vi "ControlUI_Main.vi"(5 "Splash StatusRef":refnum<vi>, 7 "Splash VI Ref":refnum<vi>, 10 "Application":refnum<class "Application.lvclass">, 11 "Main.lvclass":refnum<class "Main.lvclass">) -> ()   [LabVIEW 2019, in "Main.lvclass"]
doc: "Developed by Kevin Thompson\nkevin@thompsonengineering.net\n\nCopyright 2018\nThompson Engineering, LLC"
uses:
  Main.lvclass
  Application/Application.lvclass
  Common/DataTypes/Measurement Config--cluster.ctl
  support/Data Algorithms/subvis/DataTypes/ESR scaling--cluster.ctl
  Common/DataTypes/Acquisition Mode--cluster.ctl
  support/Data Algorithms/subvis/DataTypes/Gain control.ctl
  DataTypes/ESR values--cluster.ctl
  <vilib>/userDefined/High Color/nirio_resource_hc.ctl
  DataTypes/Control UI - AppData--cluster.ctl
  DataTypes/Settings--cluster.ctl
  DataTypes/Dependency--cluster.ctl
  Config/Config.lvclass
  DAQ_Engine/DAQ_Engine.lvclass
  Log_Engine/Log_Engine.lvclass
  DataTypes/Public Events--cluster.ctl
  Common/DataTypes/TD Async CmdMsg EventData--cluster.ctl
  Common/DataTypes/UpdateControlValue EvData--cluster.ctl
  DataTypes/ProcessingStateChg EvData--cluster.ctl
  DataTypes/ProcessingState--enum.ctl
  Common/DataTypes/InverterWaveforms--QRef.ctl
  Common/DataTypes/InverterWaveforms--cluster.ctl
  Common/DataTypes/ChannelWaveforms--cluster.ctl
  Common/DataTypes/DataProcAuxDat--Qref.ctl
  DataTypes/DataProcessAuxData--cluster.ctl
  <vilib>/TELLC/Dynamic CVT API/TD Dynamic CVT DVR--ref.ctl
  Common/DataTypes/TD GetSet ActionSelect--enum.ctl
  Main.lvclass/Main.ctl
  DAQ_Engine/DataTypes/AsynCmd_DAQ_Engine--enum.ctl
  DataTypes/PrivateAsynEv_Main--enum.ctl
  DataTypes/AsynMsg_Main--enum.ctl
  DataTypes/InverterInfo--cluster.ctl
  DataTypes/StartProcInitParams--cluster.ctl
  DataTypes/ProcessInitParams--cluster.ctl
  Common/DataTypes/DAQState--enum.ctl
  Common/DataTypes/LogState--enum.ctl
  Common/DataTypes/TDMSState--enum.ctl
  Log_Engine/Log_Engine.lvclass/Log_Engine.ctl
  DAQ_Engine/DAQ_Engine.lvclass/DAQ_Engine.ctl
  Application/DataTypes/AsynMsg_Application--enum.ctl
  Common/DataTypes/Inverter database record v2--cluster.ctl
  Common/DataTypes/inverter info v2--cluster.ctl
  Common/DataTypes/inverter gain range--cluster.ctl
  Common/DataTypes/inverter offset range--cluster.ctl
  Accessors/Get Settings.vi
  Accessors/Get PublicEvents.vi
  Accessors/Get Dependency.vi
  Accessors/Get TerminateAppEvent.vi
  Accessors/Get InvWfms-DT-QRef.vi
  Accessors/Get DPAuxData-QRef.vi
  Accessors/Get InverterLUT Dict Ref.vi
  Accessors/Get CurrInverter Record.vi
  Accessors/Set CurrInverter Record.vi
  Accessors/Get ObjData.vi
  Log_Engine/Accessors/Get PublicEvents.vi
  DAQ_Engine/Accessors/Get PublicEvents.vi
  DAQ_Engine/Accessors/Get MeasSettings.vi
  DAQ_Engine/Accessors/Get Settings.vi
  <userlib>/_OpenG.lib/comparison/comparison.llb/String Changed__ogtk.vi
  <vilib>/TELLC/SMQ/Add States to Queue using MultiLine String with vData.vi
  <userlib>/_OpenG.lib/error/error.llb/Filter Error Codes (Array)__ogtk.vi
  Common/Startup/GBL System.vi
panel:
  in  "Acqusition Mode":T1
  in  "Trigger SelectInverter Event":bool
  in  "LeftPanelTab":T2(tab)=enum."Settings"
  out "InvSelLED":bool
  in  "Selected Inverter":string[](array[string])
  in  "SelectInverter":bool
  in  "Inverter List":i32[](listbox)
  in  "Signal scaling":T3[](array[typedef])
  in  "Degassing rate\n9775":u32=3
  in  "Averaging samples\n9215":u32=480000
  in  "Data Rate 9215\n(S/s)":dbl=1200000.0 format="%#.6p"
  in  "Data Rate 9775\n(S/s)":dbl=3.0 format="%#.6p"
  out "DAQEnabled":bool=TRUE
  in  "DAQEnDis":bool
  out "LogEnabled":bool
  in  "LogEnDis":bool
  out "TDMSEnabled":bool
  in  "TDMSEnDis":bool
  in  "StopProcessing":bool caption="StopProcess"
  out "Processing":bool=TRUE
  in  "StartProcessing":bool caption="StartProcess"
  in  "UpdateDAQSettings":bool
  in  "cRIO Error\nReporting Mode":i32(ring) items=["DONTPRINT", "PRINTWARNINGS", "PRINTFATAL", "PRINTALL"]
  in  "NumPF RdsToAvg":i32=2 caption="Number PF\nReads to Avg"
  in  "ESR alarm threshhold (%)":dbl=200.0
  in  "# readings to average":i32=40
  in  "RIO Device":T4
  out "DP AuxData Size":i32
  out "InvWfmsQ DT size":i32
  in  "Inverter ID":string
  in  "toggle scrollbars":bool
  in  "toggle MainTabDbgPg":bool
  out "DAQ Running":bool=TRUE
  out "MeasSet":T5={"Data Rate 9775"=3.0, "Data Rate 9215"=1200000.0, "Samples RMS 9215"=480000, "Samples RMS 9775"=3}
  out "DAQError":bool caption="DAQ Error"
  in  "SystemError":bool
  out "Sel_PowerFactor_Data":bool=TRUE
  in  "Show_PowerFactor_Data":bool
  out "Sel_TimeSeries_Data":bool
  in  "Show_TimeSeries_Data":bool
  out "Sel_ESR_Data":bool
  in  "Show_ESR_Data":bool
  in  "MainPanelTab":T6(tab)=enum."PowerFactorData"
  in  "StoreESR BLine":bool
  in  "UseSavedESR BLine":bool
  in  "set alarm":bool
  in  "reset averaging":bool
  in  "reset alarm":bool
  in  "ESR scaling":T7[](array[typedef]) caption="ESR scaling\n(manual adjustment)" {"Offset" format="%^#_6g"; "Gain" format="%^#_6g"}
  in  "Tab Control":enum32{"DUT1", "DUT2", "DUT3", "DUT4"}(tab)
  out "ESR values 1":T8 caption="ESR values" {"Scaled & avgd ESR" format="%_4e"; "Max ESR" format="%_4e"; "Raw  ESR" format="%.3e"}
  out "Equivalent Series Resistance (ESR) 1":T9(graph)
  in  "MinCurrThreshold 1":dbl=1.5 caption="Minimum Current\nThreshold (A)" format="%.8f"
  in  "Sensor Type 1":i32(ring)
  in  "Sensor Type 2":i32(ring)
  in  "MinCurrThreshold 2":dbl=1.5 caption="Minimum Current\nThreshold (A)" format="%.8f"
  out "ESR values 2":T8 caption="ESR values" {"Scaled & avgd ESR" format="%_4e"; "Max ESR" format="%_4e"; "Raw  ESR" format="%.3e"}
  out "Equivalent Series Resistance (ESR) 2":T9(graph)
  in  "Sensor Type 3":i32(ring)
  in  "MinCurrThreshold 3":dbl=1.5 caption="Minimum Current\nThreshold (A)" format="%.8f"
  out "ESR values 3":T8 caption="ESR values" {"Scaled & avgd ESR" format="%_4e"; "Max ESR" format="%_4e"; "Raw  ESR" format="%.3e"}
  out "Equivalent Series Resistance (ESR) 3":T9(graph)
  in  "Sensor Type 4":i32(ring)
  in  "MinCurrThreshold 4":dbl=1.5 caption="Minimum Current\nThreshold (A)" format="%.8f"
  out "ESR values 4":T8 caption="ESR values" {"Scaled & avgd ESR" format="%_4e"; "Max ESR" format="%_4e"; "Raw  ESR" format="%.3e"}
  out "Equivalent Series Resistance (ESR) 4":T9(graph)
  out "Iout 60Hz":waveform(dbl)[](graph)
  out "Iout ripple":waveform(dbl)[](graph)
  out "Iin ripple":waveform(dbl)[](graph)
  out "DUT4 I-V":waveform(dbl)[](graph) caption="DUT 4"
  out "DUT3 power data":T10 caption="Phase 1" {"Vout (RMS)" format="%0.2f"; "Iout (RMS)" format="%0.2f"; "PF" format="%.3g"}
  out "DUT2 power data":T10 caption="Phase 1" {"Vout (RMS)" format="%0.2f"; "Iout (RMS)" format="%0.2f"; "PF" format="%.3g"}
  out "DUT3 I-V":waveform(dbl)[](graph) caption="DUT 3"
  out "DUT2 I-V":waveform(dbl)[](graph) caption="DUT 2"
  out "DUT1 I-V":waveform(dbl)[](graph) caption="DUT 1"
  out "DUT1 power data":T10 caption="Phase 1" {"Vout (RMS)" format="%0.2f"; "Iout (RMS)" format="%0.2f"; "PF" format="%.3g"}
  in  "Dummy Vrms":dbl format="%.2g"
  in  "UseDummyVrms":bool
  out "DUT4 power data":T10 caption="Phase 1" {"Vout (RMS)" format="%0.2f"; "Iout (RMS)" format="%0.2f"; "PF" format="%.3g"}
  in  "Page2Pg_button":bool
  in  "SettingsPg_button":bool
  in  "DataPg_button":bool
  in  "ConfigPg_button":bool
  in  "Exit":bool
  in  "TitleBar AppVerText":string="v2.0.2 build-003"
  in  "TitleBar Text":string="INVERTER   HEALTH   SCANNER   SYSTEM"
  in  "TitleBar":bool
  in  "StatusMsg":string caption="Status"
  in  "process sync":refnum<notifier>
  # "click to reset"
  # "Run Time Data Panel"
  # "Inverter Selection"
  # "right-click to open table editor"
  # "Configuration Panel"
  # "Gain"
  # "Offset"
  # "Iin ripple"
  # "Iout ripple"
  # "Iout 60Hz"
  # "Vout 60"
  # "Settings Panel"
  # "Ripple Current"
  # "RMS & Power Factor"
  # "ESR Data"
  # "Gain"
  # "Offset"
  # "Time Series Data"
  # "DUT 1"
  # "DUT 2"
  # "DUT 3"
  # "DUT 4"
  # "Power Factor Data - Phase Current and Voltage"
  # "DUT 3"
  # "DUT 2"
  # "DUT 1"
  # "Current (A)"
  # "Voltage (V)"
  # "DUT 4"
  # "Debug Page"
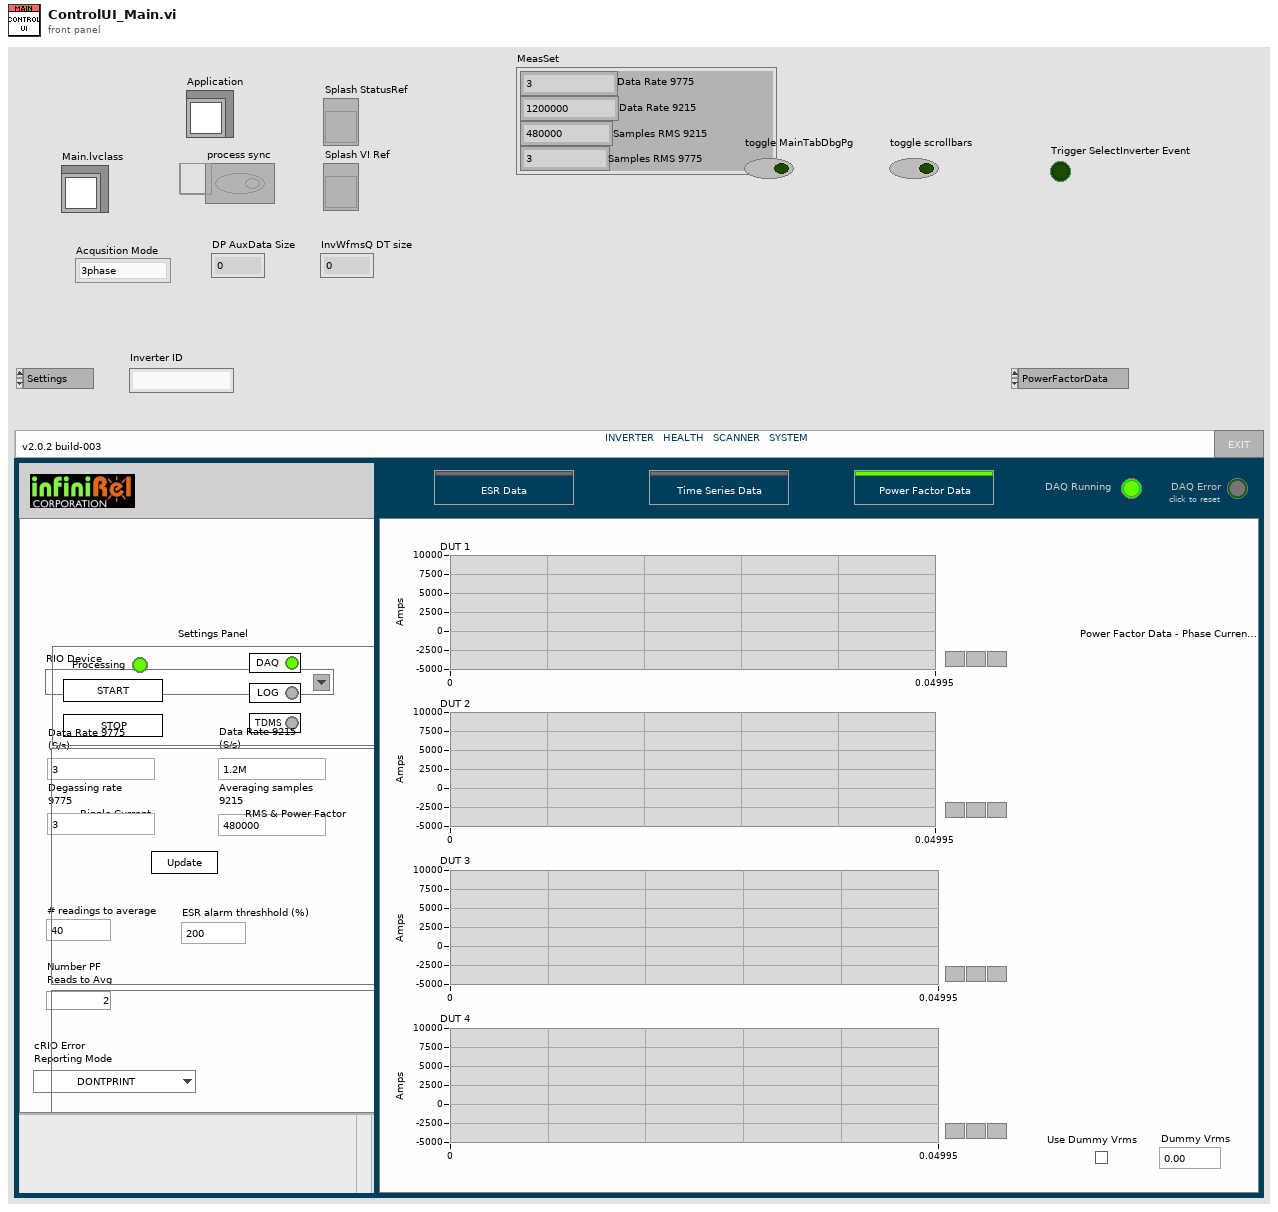
[diagram p1: front panel]
types:
  T1 = typedef "Acquisition Mode--cluster.ctl" = enum16{"3phase", "Single"}
  T2 = enum32{"Data", "InverterSel", "Config", "Settings"}
  T3 = typedef "Main.lvclass/Gain control.ctl" = cluster{"Iin ripple gain":dbl, "Iout ripple gain":dbl, "Iout 60Hz gain ":dbl, "Vout 60Hz gain ":dbl, "Iin ripple offest":dbl, "Iout ripple offset":dbl, "Iout 60Hz offset":dbl, "Vout 60Hz offset":dbl}
  T4 = typedef "nirio_resource_hc.ctl" = tag
  T5 = typedef "Measurement Config--cluster.ctl" = cluster{"Data Rate 9775":dbl, "Data Rate 9215":dbl, "Samples RMS 9215":u32, "Samples RMS 9775":u32}
  T6 = enum32{"ESRData", "TimeSeriesData", "PowerFactorData", "DebugPage"}
  T7 = typedef "Main.lvclass/ESR scaling--cluster.ctl" = cluster{"Gain":dbl, "Offset":dbl}
  T8 = typedef "Main.lvclass/ESR values--cluster.ctl" = cluster{"Inverter State":string, "Raw  ESR":dbl, "Max ESR":dbl, "Scaled & avgd ESR":dbl, "Inverter ESR status":bool}
  T9 = cluster{"ESR Baseline":dbl, "Alarm threshhold (%)":dbl, "Avg value":dbl}
  T10 = cluster{"PF":dbl, "Iout (RMS)":dbl, "Vout (RMS) ":dbl, "Power (W)":dbl}
  T11 = typedef "Main.lvclass/ProcessingState--enum.ctl" = enum16{"Idle", "Starting", "Running", "Done", "Error"}
  T12 = typedef "TD GetSet ActionSelect--enum.ctl" = enum16{"Init", "Get", "Set"}
  T13 = typedef "Main.lvclass/Control UI - AppData--cluster.ctl" = cluster{"Core":cluster{"Current VI Reference":refnum<vi>, "Close Panel on Exit?":bool}, "SMQ":refnum<queue>, "Initialized?":bool, "Self Reference":refnum<class "Main.lvclass">, "Simulation?":bool, "process sync":refnum<notifier>, "vData":variant, "Settings":T14, "Dependency":T15, "Public Events":T16, "Splash StatusRef":refnum<vi>, "Splash VI Ref":refnum<vi>, "RunTimeSystem?":bool, "StatusMsg Ref":refnum<vi>, "AppTerminateEv":refnum<user-event>, "MenuRef":refnum<k9>, "DAQEnabled":bool, "LoggingEnabled":bool, "TDMS Enabled":bool, "Application":refnum<class "Application.lvclass">, "InvWfmsQ-DT":T17, "DPAuxDataQ":T18, "ProcessingState":T11, "DisplayLoopInterval":u32, "MenuBarShown?":bool, "InverterNames[]":string[], "InverterLUT Dict":T19}
  T14 = typedef "Main.lvclass/Settings--cluster.ctl" = cluster{"Simulation":bool, "Signal scaling":T3[], "ESR scaling":T7[], "num readings to average":i32[], "ESR alarm threshhold (%)":i32[], "UseDummyVrms":bool, "Dummy Vrms":dbl, "Inverter Database File":path, "default Inverter (name)":string[], "Minimum Current Threshold ":dbl[], "Sensors Database File":path, "default Sensors (name)":string[]}
  T15 = typedef "Main.lvclass/Dependency--cluster.ctl" = cluster{"Config":refnum<class "Config.lvclass">, "DAQ":refnum<class "DAQ_Engine.lvclass">, "Log_Engine":refnum<class "Log_Engine.lvclass">}
  T16 = typedef "Main.lvclass/Public Events--cluster.ctl" = cluster{"Main.AsyncCmd Event":refnum<user-event>, "Main.AsyncMsg Event":refnum<user-event>, "stop process":refnum<user-event>, "UpdateControlValue Ev":refnum<user-event>, "ProcessingStateChg Ev":refnum<user-event>}
  T17 = typedef "InverterWaveforms--QRef.ctl" = refnum<queue>
  T18 = typedef "DataProcAuxDat--Qref.ctl" = refnum<queue>
  T19 = typedef "TD Dynamic CVT DVR--ref.ctl" = refnum<data-value>
  T20 = cluster{"AvgPF":dbl, "IoutRMS_A":dbl, "VoutRMS_V":dbl, "Power_W":dbl}
  T21 = typedef "DataProcessAuxData--cluster.ctl" = cluster{"Time Stamp":timestamp, "Raw ESR sum":dbl, "Inv 1 ON?":bool, "Average scaled ESR sum":dbl, "Inv 1 over threshold?":bool, "Inv 1 ESR":cluster{"ESR Baseline":dbl, "Alarm threshhold (%)":dbl, "Avg value":dbl}, "Max ESR":dbl}
  T22 = cluster{"Inverter 1 state: ":string, "Raw ESR sum":dbl, "Max ESR":dbl, "Average scaled ESR sum":dbl, "Inv 1 over threshold?":bool}
  T23 = typedef "InverterWaveforms--cluster.ctl" = T24[]
  T24 = typedef "ChannelWaveforms--cluster.ctl" = cluster{"Iin ripple ":waveform(dbl), "Iout ripple ":waveform(dbl), "Iout 60Hz":waveform(dbl), "Vout 60Hz":waveform(dbl)}
  T25 = typedef "DAQ_Engine.lvclass/AsynCmd_DAQ_Engine--enum.ctl" = enum16{"DAQ.EnableDAQ", "DAQ.ClearDAQError", "DAQ.SetMeasConfig", "DAQ.SetAcqMode", "DAQ.SetErrorReporting"}
  T26 = typedef "Main.lvclass/PrivateAsynEv_Main--enum.ctl" = enum16{"PrivMain.UpdateMeasSettings", "PrivMain.UpdateAcqMode", "PrivMain.UpdateDAQState", "PrivMain.UpdateLogState", "PrivMain.UpdateTDMSState", "PrivMain.UpdateProcessingState", "PrivMain.Stop&Terminate", "PrivMain.CurrInverterUpdated", "PrivMain.UpdateStoreUseESRBaseline", "PrivMain.SetUnsetAlarm&ESRBLine", "PrivMain.ResetAveraging"}
  T27 = typedef "Main.lvclass/AsynMsg_Main--enum.ctl" = enum16{"Main.CurrInverterUpdated"}
  T28 = typedef "Main.lvclass/StartProcInitParams--cluster.ctl" = cluster{"InverterInfo":T29[], "ProcessInitParams":T30[]}
  T29 = typedef "InverterInfo--cluster.ctl" = cluster{"Inverter ID":string}
  T30 = typedef "Main.lvclass/ProcessInitParams--cluster.ctl" = cluster{"MinCurrThreshold":dbl, "NumPF RdsToAvg":i32, "ESR alarm threshhold (%)":dbl, "# readings to average":i32}
  T31 = typedef "DAQState--enum.ctl" = enum16{"Unknown", "Stopped", "Running", "Error"}
  T32 = cluster{"VoltageDyn":dbl, "CurrentDyn":dbl, "MotorV SP":dbl}[]
  T33 = enum32{"invalid app kind", "Development System", "Run Time System", "Student Edition", "Embedded LabVIEW", "Evaluation", "Custom"}
  T34 = typedef "Application.lvclass/AsynMsg_Application--enum.ctl" = enum16{"Application.AppClassReference"}
  T35 = enum16{"Left Button", "Center Button", "Right Button", "Window Close"}
  T36 = enum32{"Invalid", "Standard", "Closed", "Hidden", "Minimized", "Maximized"}
  T37 = enum32{"Invalid", "Default", "Floating", "Floating/Auto-Hide", "Modal"}
  T38 = typedef "Inverter database record v2--cluster.ctl" = cluster{"name":string, "last updated":timestamp, "type":string, "inverter Info":T39, "gain range":T40, "offset range":T41, "gain actual":dbl, "offset actual":dbl, "power level":dbl, "minimum current":dbl, "resistance single phase":dbl, "resistance 3 phase":dbl, "set flag":u16}
  T39 = typedef "inverter info v2--cluster.ctl" = cluster{"manufacturer":string, "model":string, "product":string, "serial":string, "power class":string, "year manf":string}
  T40 = typedef "inverter gain range--cluster.ctl" = cluster{"gain max":dbl, "gain min":dbl, "gain increment":dbl}
  T41 = typedef "inverter offset range--cluster.ctl" = cluster{"offset max":dbl, "offset min":dbl, "offset increment":dbl}
  T42 = typedef "Config.lvclass/Config Settings.ctl" = cluster{"Application Settings":T43, "Main Settings":T14, "DAQ Settings":T44, "LogEngine Settings":T45}
  T43 = typedef "Application.lvclass/Settings--cluster.ctl" = cluster{"Simulation":bool}
  T44 = typedef "DAQ_Engine.lvclass/Settings--cluster.ctl" = cluster{"Simulation":bool, "Initial ErrReporting setting":i32, "Initial Measurement settings":T5, "Acquisition mode":T1, "DemoMode":bool, "RIO Device":string}
  T45 = typedef "Log_Engine.lvclass/Settings--cluster.ctl" = cluster{"Simulation":bool, "TDMS_FolderPath":string, "CSV_FolderPath":string, "TDMS_FileName_Prefix":string, "CSV_FileName_Prefix":string, "TDMS_LogDuration(s)":dbl, "CSV_LogDuration(s)":dbl}
  T46 = typedef "TD Pathnames--cluster.ctl" = cluster{"RunTimeSys?":bool, "AppFolder":path, "ExecutablePath":path, "ConfigFolder":path, "DataLogFolder":path, "SystemLogFolder":path, "SeqFolder":path, "MainStartupPathname":path, "MainUIPathname":path, "SystemEventsFile":path, "SeqEventsFile":path, "Config SettingsFile":path, "DAQ IOConfigFile":path, "SystemSimulation":bool}
  T47 = typedef "DAQ_Engine.lvclass/DAQStateEvData--cluster.ctl" = cluster{"DAQState":T31, "vData":variant}
  T48 = typedef "LogState--enum.ctl" = enum16{"Unknown", "Stopped", "Running", "Error"}
  T49 = typedef "Log_Engine.lvclass/LogStateEvData--cluster.ctl" = cluster{"LogState":T48, "vData":variant}
  T50 = typedef "TDMSState--enum.ctl" = enum16{"Unknown", "Stopped", "Running", "Error"}
  T51 = typedef "Log_Engine.lvclass/TDMSStateEvData--cluster.ctl" = cluster{"TDMSState":T50, "vData":variant}
  T52 = typedef "Main.lvclass/AsynCmd_Main--enum.ctl" = enum16{"Main.StartProcessing", "Main.StopProcessing", "Main.RefreshInverterList"}
  T53 = typedef "Main.lvclass/ObjData--cluster.ctl" = cluster{"Settings":T14, "Public Events":T16, "Dependency":T15, "ReadData-placeholder":T54, "VISA-placeholder":refnum<visa-resource-name>, "InverterWaveformsQ":T17, "Application.TerminateProcess Event":refnum<user-event>, "RawDaqDataQ":T55, "MeasSettings":T5, "InverterDataAcqMode":T1, "DAQState Data":T47, "Private Events":T56, "InvWfmsQ-DT":T17, "DPAuxDataQ":T18, "ProcessingState":T11, "InverterInfo":T29, "CurrInverters":T38[], "InverterLUT Dict":T19, "ESR Chart Ref":refnum<vi>[], "StoreESR BLine Ref":refnum<vi>, "UseSavedESR BLine Ref":refnum<vi>, "CurrSensor":T57, "SensorLUT Dict":T19}
  T54 = typedef "Main.lvclass/Read Data--cluster.ctl" = cluster{"Data":dbl}
  T55 = typedef "RawDAQDataQRef--cluster.ctl" = refnum<queue>
  T56 = typedef "Main.lvclass/Private Events--cluster.ctl" = cluster{"PrivateAsync Ev":refnum<user-event>}
  T57 = typedef "Sensor LUT--cluster.ctl" = T58[]
  T58 = typedef "Sensor database record--cluster.ctl" = cluster{"name":string, "last updated":timestamp, "manufacturer":string, "model":string, "Sensitivity index":dbl, "Sensor Ranges":T59}
  T59 = typedef "Sensor ranges--cluster.ctl" = cluster{"Max.VOut.RMS (V)":dbl, "Max.Out.Peak (V)":dbl, "Sensitivity (mV/A)":dbl, "Max.IOut.RMS(A)":dbl, "Min.IOut.RMS(A)":dbl}
  T60 = typedef "DAQ_Engine.lvclass/Public Events--cluster.ctl" = cluster{"DAQ_Engine.AsyncCmd Event":refnum<user-event>, "DAQ_Engine.AsyncMsg Event":refnum<user-event>, "stop process":refnum<user-event>, "DAQ_Engine.DAQStateChg Ev":refnum<user-event>, "DAQ_Engine.MeasSettingsChg Ev":refnum<user-event>, "DAQ_Engine.AcqModeChg Ev":refnum<user-event>}
  T61 = typedef "Log_Engine.lvclass/Public Events--cluster.ctl" = cluster{"Log_Engine.AsyncCmd Event":refnum<user-event>, "Log_Engine.AsyncMsg Event":refnum<user-event>, "stop process":refnum<user-event>, "Log_Engine.LogStateChg Ev":refnum<user-event>, "Log_Engine.TDMSStateChg Ev":refnum<user-event>}
  T62 = cluster{"Current VI Reference":refnum<vi>, "Close Panel on Exit?":bool}
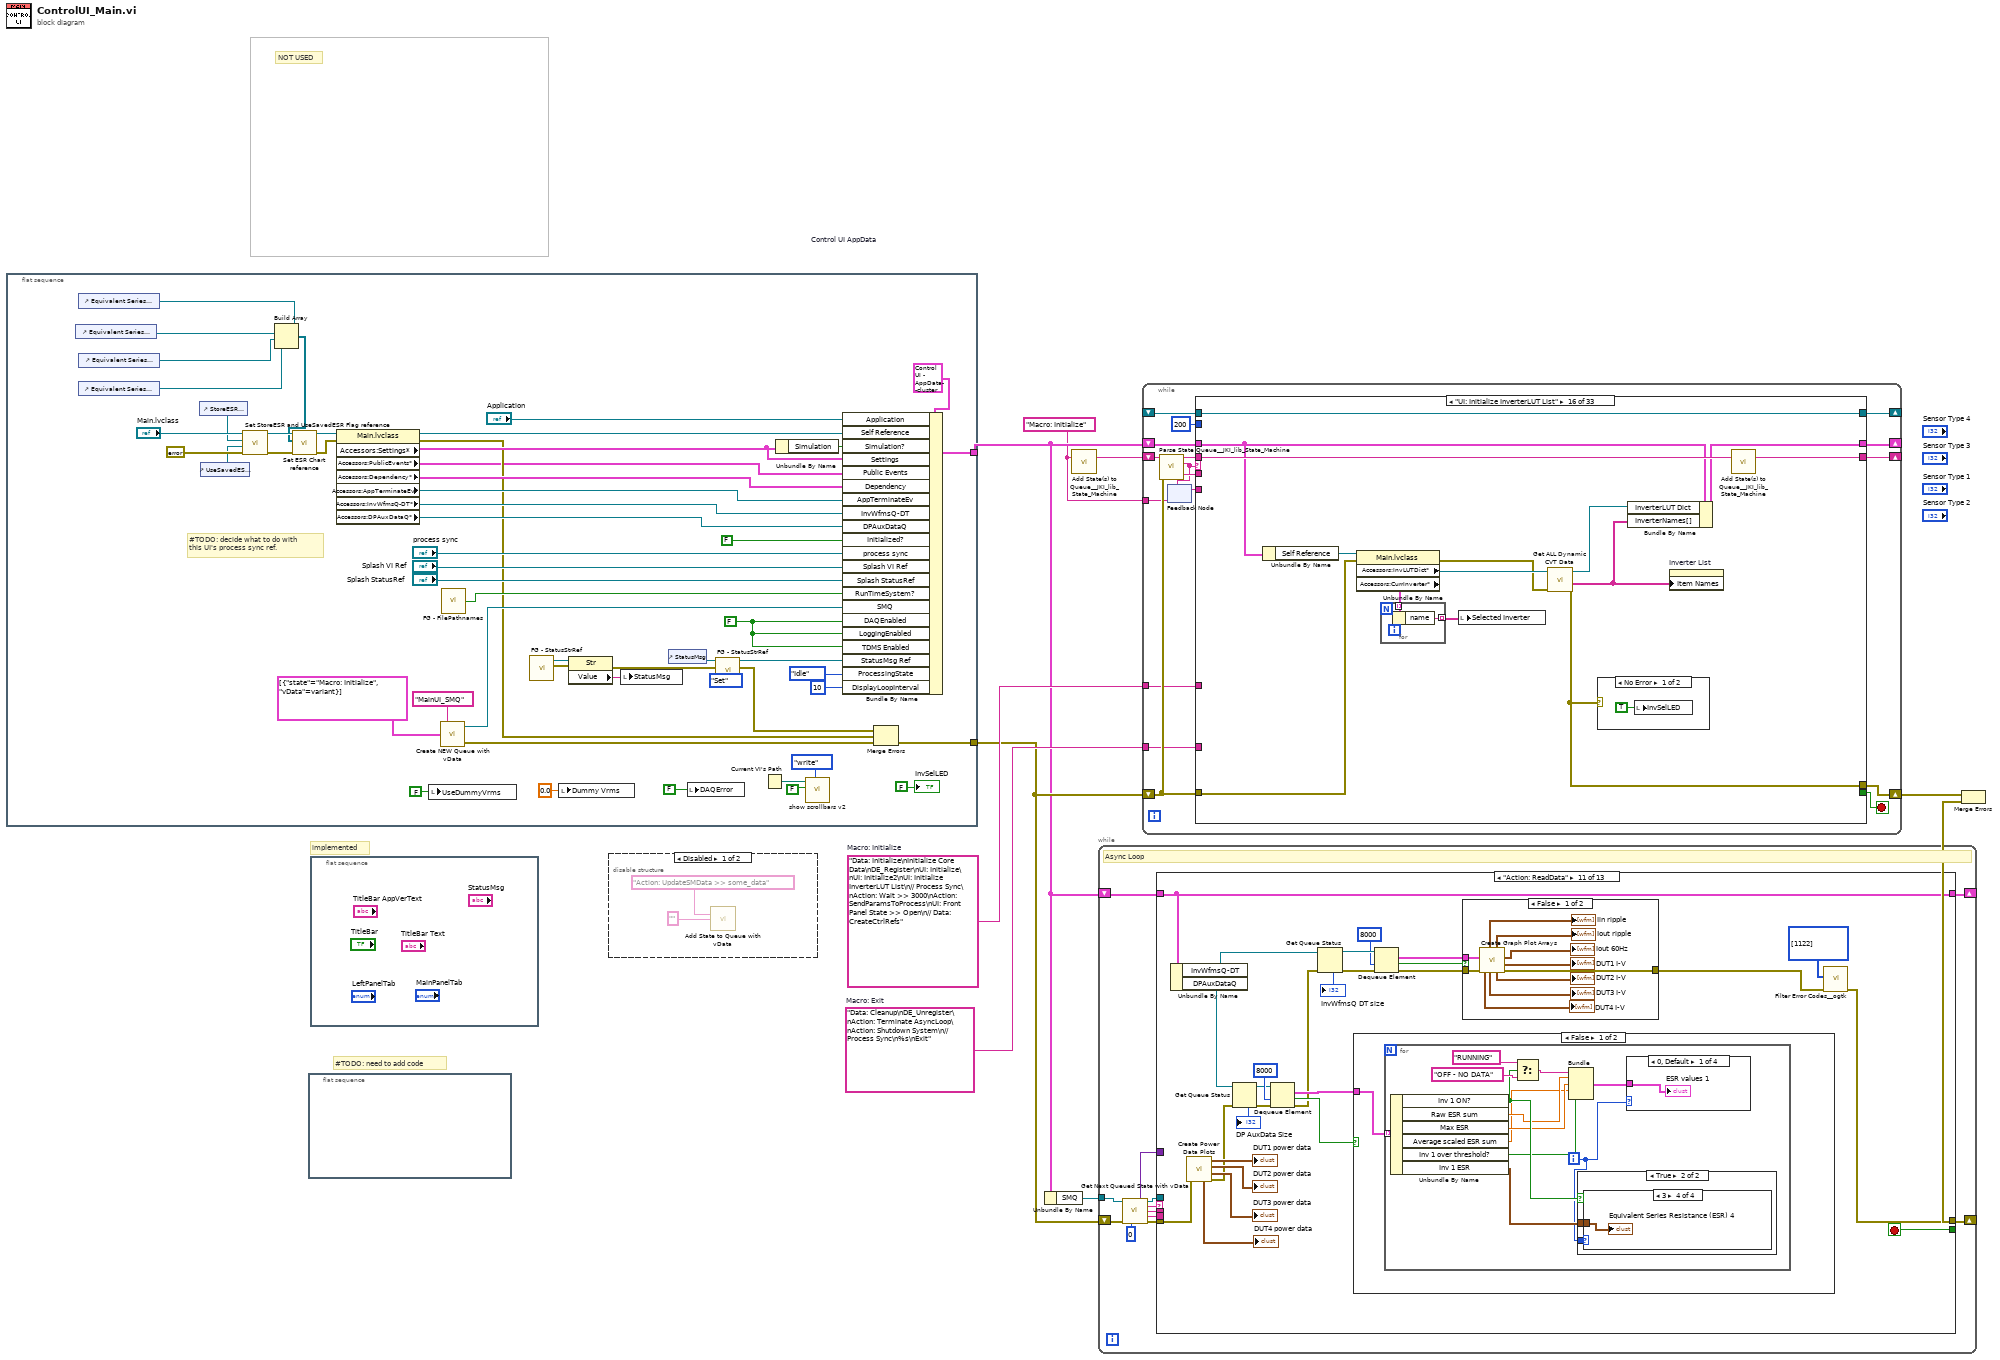
[diagram p0: block diagram]
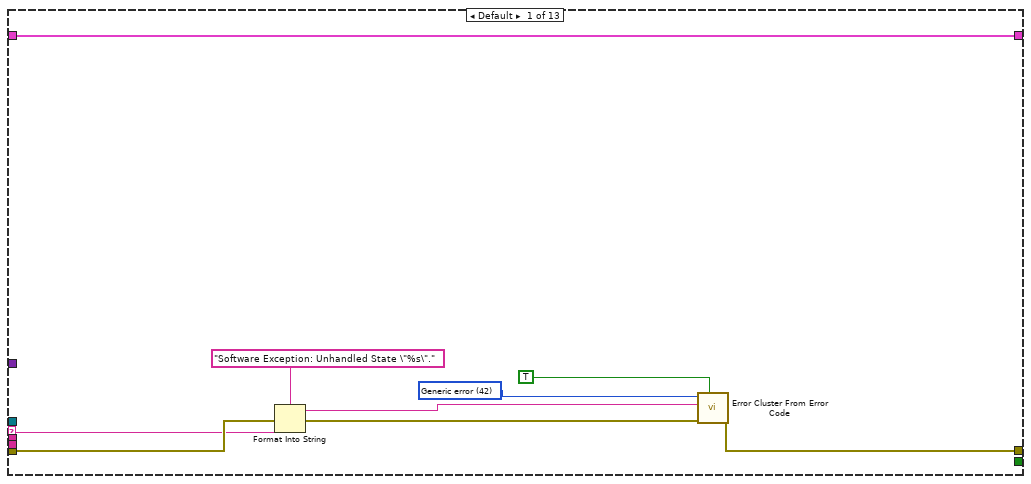
[diagram p3: hidden frame]
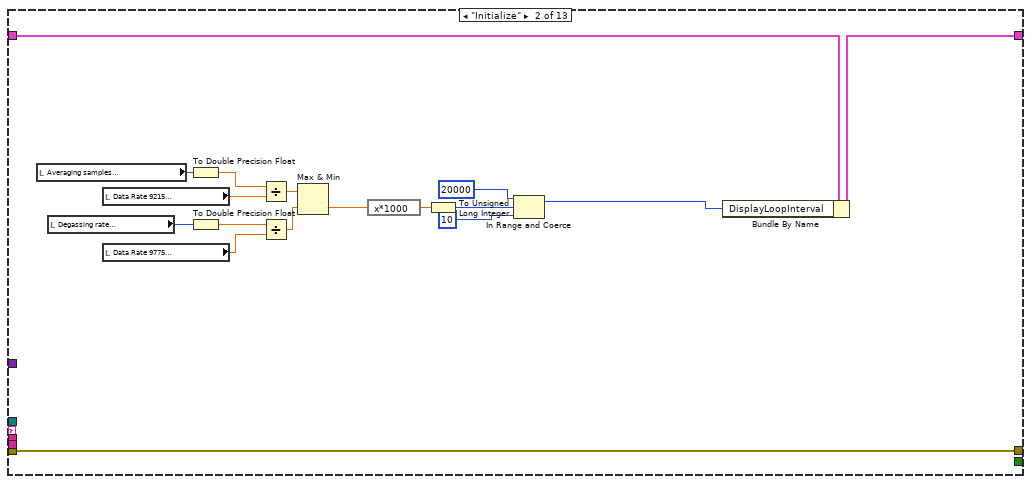
[diagram p4: hidden frame]
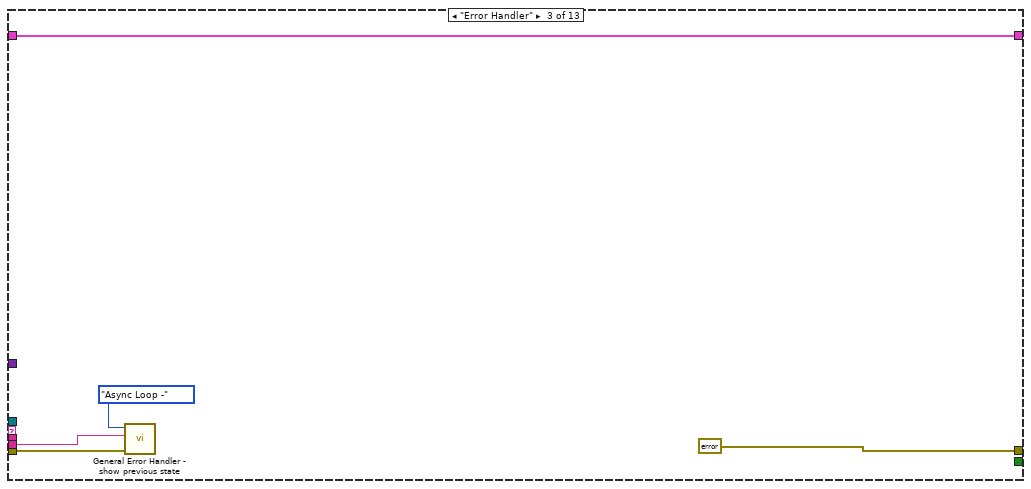
[diagram p5: hidden frame]
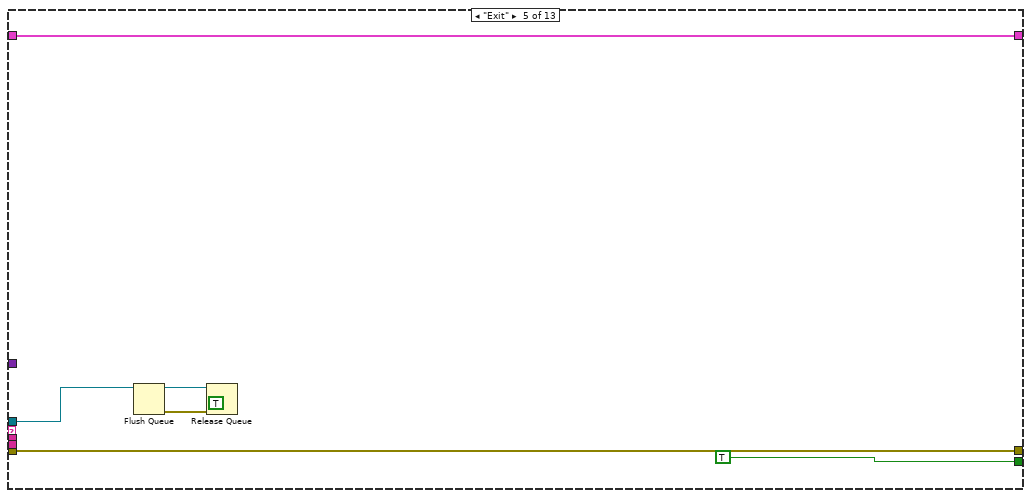
[diagram p7: hidden frame]
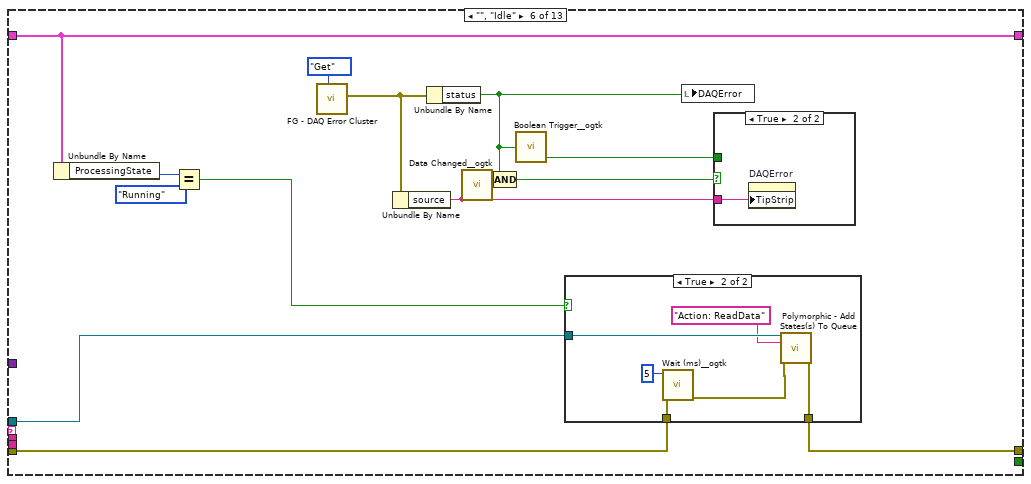
[diagram p8: hidden frame]
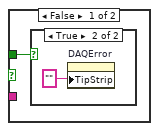
[diagram p9: hidden frame]
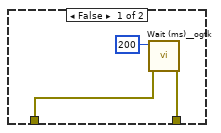
[diagram p11: hidden frame]
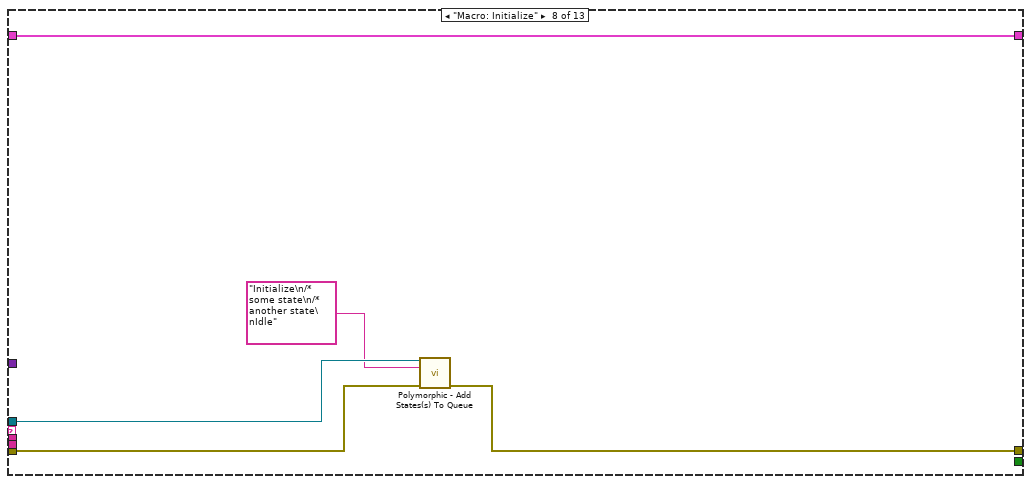
[diagram p13: hidden frame]
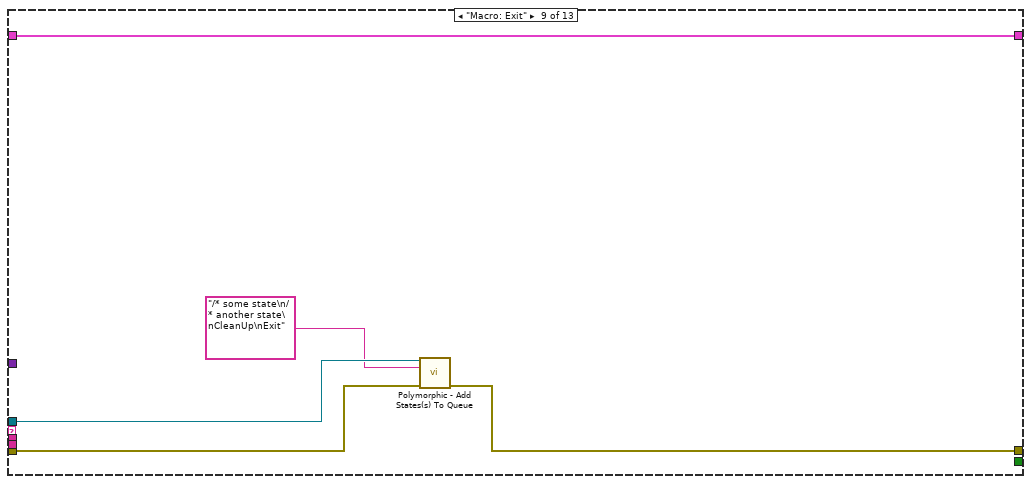
[diagram p14: hidden frame]
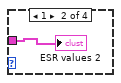
[diagram p16: hidden frame]
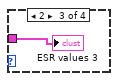
[diagram p17: hidden frame]
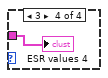
[diagram p18: hidden frame]
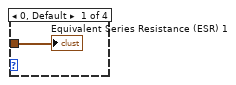
[diagram p20: hidden frame]
diagram:
  w7 = "Data: Cleanup\nDE_Unregister\nAction: Terminate AsyncLoop\nAction: Shutdown System\n// Process Sync\n%s\nExit"  # Macro: Exit
  w8 = "Data: Initialize\nInitialize Core Data\nDE_Register\nUI: Initialize\nUI: Initialize2\nUI: Initialize InverterLUT List\n// Process Sync\nAction: Wait >> 3000\nAction: SendParamsToProcess\nUI: Front Panel State >> Open\n// Data: CreateCtrlRefs"  # Macro: Initialize
  w1 = "Macro: Initialize"
  # "implemented"
  # "#TODO: need to add code"
  # "NOT USED"
  n1 = flat-sequence {
    tunnel: [w62] -> w4
    tunnel: [w47] -> w6
    frame #0 {
      w33 = FALSE
      w54 = T13 {"Core"={"Current VI Reference"=refnum, "Close Panel on Exit?"=FALSE}, "SMQ"=refnum, "Initialized?"=FALSE, "Self Reference"=refnum, "Simulation?"=FALSE, "process sync"=refnum, "vData"=variant, "Settings"={"Simulation"=FALSE, "Signal scaling"=[], "ESR scaling"=[], "num readings to average"=[], "ESR alarm threshhold (%)"=[], "UseDummyVrms"=FALSE, "Dummy Vrms"=0.0, "Inverter Database File"=path "", "default Inverter (name)"=[], "Minimum Current Threshold "=[], "Sensors Database File"=path "", "default Sensors (name)"=[]}, "Dependency"={"Config"=refnum, "DAQ"=refnum, "Log_Engine"=refnum}, "Public Events"={"Main.AsyncCmd Event"=refnum, "Main.AsyncMsg Event"=refnum, "stop process"=refnum, "UpdateControlValue Ev"=refnum, "ProcessingStateChg Ev"=refnum}, "Splash StatusRef"=refnum, "Splash VI Ref"=refnum, "RunTimeSystem?"=FALSE, "StatusMsg Ref"=refnum, "AppTerminateEv"=refnum, "MenuRef"=refnum, "DAQEnabled"=FALSE, "LoggingEnabled"=FALSE, "TDMS Enabled"=FALSE, "Application"=refnum, "InvWfmsQ-DT"=refnum, "DPAuxDataQ"=refnum, "ProcessingState"=enum."Idle", "DisplayLoopInterval"=0, "MenuBarShown?"=FALSE, "InverterNames[]"=[], "InverterLUT Dict"=refnum}  # Control UI AppData
      # "#TODO: decide what to do with\nthis UI's process sync ref."
      n2 = control-ref of="Equivalent Series Resistance (ESR) 2"() -> (w12:refnum<vi>)
      n3 = control-ref of="Equivalent Series Resistance (ESR) 1"() -> (w14:refnum<vi>)
      n4 = control-ref of="Equivalent Series Resistance (ESR) 4"() -> (w10:refnum<vi>)
      n5 = control-ref of="Equivalent Series Resistance (ESR) 3"() -> (w11:refnum<vi>)
      n6 = control-ref of="StoreESR BLine"() -> (w15:refnum<vi>)
      n7 = control-ref of="UseSavedESR BLine"() -> (w16:refnum<vi>)
      n8 = call "Set StoreESR and UseSavedESR Flag reference.vi"("error in (no error)"=errorcluster {"status"=FALSE, "code"=0, "source"=""} ("error constant"), "UseSavedESR BLine Ref"=w16, "StoreESR BLine Ref"=w15, "Main in"="Main.lvclass") -> ("error out"=w19:errorcluster, "Main out"=w20:refnum<class "Main.lvclass">)  [unwired: 6 in]
      n9 = Build Array(w14, w12, w11, w10) -> (w13:refnum<vi>[])
      n10 = call "Set ESR Chart reference.vi"("error in (no error)"=w19, "ESR Chart Ref"=w13, "Main in"=w20) -> ("error out"=w17:errorcluster, "Main out"=w22:refnum<class "Main.lvclass">)  [unwired: 7 in]
      n11 = property class="Main.lvclass"(reference=w22, error in=w17) -> (reference out=w25:refnum<class "Main.lvclass">, error out=w26:errorcluster, "Accessors:Settings*"=w56:T14, "Accessors:PublicEvents*"=w24:T16, "Accessors:Dependency*"=w58:T15, "Accessors:AppTerminateEv*"=w53:refnum<user-event>, "Accessors:InvWfmsQ-DT*"=w32:T17, "Accessors:DPAuxDataQ*"=w31:T18)
      n12 = local write "UseDummyVrms"(FALSE ("UseDummyVrms")) -> ()
      n13 = call <vilib>:"Create NEW Queue with vData.vi"("Initial States"=cluster{"state":string, "vData":variant}[] [{"state"="Macro: Initialize", "vData"=variant}], "Name (SMQ)"="MainUI_SMQ") -> ("error out"=w48:errorcluster, "queue out"=w52:refnum<queue>)  [unwired: 2 in]
      n14 = call "FG - FilePathnames.vi"() -> ("RunTimeSys?"=w49:bool)  [unwired: 4 in, 1 out]
      n15 = call "FG - StatusStrRef.vi"() -> ("StatusStr Ref out"=w46:refnum<vi>, "error out"=w45:errorcluster)  [unwired: 9 in]
      n16 = local write "Dummy Vrms"(0.0 ("Dummy Vrms")) -> ()
      n17 = property class="Str"(reference=w46, error in=w45) -> (error out=w44:errorcluster, "Value"=w43:string)  [unwired: 1 out]
      n18 = local write "StatusMsg"(w43) -> ()
      n19 = control-ref of="StatusMsg"() -> (w42:refnum<vi>)
      n20 = local write "DAQError"(FALSE ("SystemError")) -> ()
      n21 = call "FG - StatusStrRef.vi"("StatusStr Ref in"=w42, "error in (no error)"=w44, "action (Get)"=TD_GetSet_ActionSelect--enum."Set") -> ("StatusStr Ref out"=w40:refnum<vi>, "error out"=w39:errorcluster)  [unwired: 6 in]
      n22 = Current VI's Path() -> (path=w38:path)
      n23 = Unbundle By Name(w56) -> ("Simulation"=w57:bool)
      n24 = call <vilib>:"show scrollbars v2.vi"("mode (read)"=enum16{"read", "write", "toggle"}."write", "ShowScrollbars?"=FALSE, "vi path"=w38) -> ()  [unwired: 4 in, 2 out]
      n25 = Bundle By Name(cluster=w54, "Application"="Application", "Self Reference"=w25, "Simulation?"=w57, "Settings"=w56, "Public Events"=w24, "Dependency"=w58, "AppTerminateEv"=w53, "InvWfmsQ-DT"=w32, "DPAuxDataQ"=w31, "Initialized?"=FALSE, "process sync"="process sync", "Splash VI Ref"="Splash VI Ref", "Splash StatusRef"="Splash StatusRef", "RunTimeSystem?"=w49, "SMQ"=w52, "DAQEnabled"=w33, "LoggingEnabled"=w33, "TDMS Enabled"=w33, "StatusMsg Ref"=w40, "ProcessingState"=ProcessingState--enum."Idle", "DisplayLoopInterval"=u32 10) -> (w62:T13)
      n26 = Merge Errors(w39, w26, w48) -> (w47:errorcluster)
      "InvSelLED" <- FALSE ("InvSelLED")
    }
  }
  n27 = flat-sequence {
    frame #0 {
    }
  }
  n28 = flat-sequence {
    frame #0 {
    }
  }
  n29 = disable-structure shown="Disabled" {
    frame Disabled {
      n30 = call <vilib>:"Add State to Queue with vData.vi"("state in"="Action: UpdateSMData >> some_data", "vData (\"\")"="") -> ()  [unwired: 10 in, 4 out]
    }
    frame Enabled {
    }
  }
  n31 = Unbundle By Name(w4) -> ("SMQ"=w5:refnum<queue>)
  n32 = call <vilib>:"Add State(s) to Queue__JKI_lib_State_Machine.vi"("State(s) in (\"\")"=w1) -> ("States Out"=w9:string)  [unwired: 14 in]
  n33 = while {
    shift-right: [w74] -> w2
    shift-left: w6 -> [w76]
    tunnel: w5 -> [w72]
    shift-right: [w70] -> _
    shift-left: w4 -> [w71]
    stop <- w65 stop-if-true
    # "Async Loop"
    n34 = call <vilib>:"Get Next Queued State with vData.vi"("queue in"=w72, "error in (no error)"=w76, "timeout (100)"=0) -> ("vData out"=w69:variant, "queue out"=w73:refnum<queue>, "Next State"=w77:string, "queued msg"=w67:string, "Prev State"=w66:string, "error out"=w75:errorcluster)  [unwired: 6 in, 1 out]
    n35 = case shown="\"Action: ReadData\"" w77 {
      tunnel: w73 -> [_ _ _ _ w111 w130 _ w149 w154 _ _ _ w231]
      tunnel: w67 -> [_ _ _ _ _ _ _ _ _ _ _ w220 w233]
      selector: w77 -> [w78 _ _ _ _ _ _ _ _ _ _ _ _]
      tunnel: w75 -> [w80 w103 w105 w110 w117 w128 w145 w148 w153 w157 w176 w219 w228]
      tunnel: [w79 w103 errorcluster {"status"=FALSE, "code"=0, "source"=""} ("error constant") w110 w117 w131 w145 w147 w152 w157 w160 w222 w227] -> w74
      tunnel: w71 -> [w86 w101 w108 w109 w116 w129 w144 w150 w155 w156 w183 w225 w230]
      tunnel: [w86 w102 w108 w109 w116 w129 w144 w150 w155 w156 w183 w225 w229] -> w70
      tunnel: w69 -> [_ _ _ _ _ _ _ _ _ _ _ _ w232]
      tunnel: w66 -> [_ _ w104 _ _ _ _ _ _ _ _ _ _]
      tunnel: [_ _ _ _ TRUE _ _ _ _ _ _ _ _] -> w65
      frame Default {
        w82 = 42 items=["No error", "Argument error", "Memory is full", "Out of zone", "End of file", "File already open", "Generic file I/O error", "File not found", "File permission error", "Disk is full", "Duplicate path", "Too many files open", "System feature not enabled", "Resource file not found", "Cannot add resource", "Resource not found", "Image not found", "Image memory error", "Pen does not exist", "Config type invalid", "Config token not found", "Config parse error", "Config memory error", "Bad external code format", "Bad external code offset", "External code not present", "Null window", "Destroy window error", "Null menu", "Print aborted", "Bad print record", "Print driver error", "Windows error during printing", "Memory error during printing", "Print dialog error", "Generic print error", "Invalid device refnum", "Device not found", "Device parameter error", "Device unit error", "Cannot open device", "Device call aborted", "Generic error", "Cancelled by user", "Object ID too low", "Object ID too high", "Object not in heap", "Unknown heap", "Unknown object (invalid DefProc)", "Unknown object (DefProc not in table)", "Message out of range", "Invalid (null) method", "Unknown message", "Manager call not supported", "Bad address", "Network operation in progress", "Network operation timed out", "Connection is busy", "Network attribute not supported", "Network error", "Address in use", "System out of memory", "Connection aborted", "Connection refused", "Not connected", "Already connected", "Connection closed", "Initialization error (interapplication manager)", "Bad occurrence", "Wait on unbound occurrence handler", "Occurrence queue overflow", "Datalog type conflict", "Unused", "Unrecognized type (interapplication manager)", "Memory corrupt", "Failed to make temporary DLL", "Old CIN version", "Drag socket not found", "Failed to load drop-object", "Failed to register OLE object", "Failed to release OLE object", "Format specifier type mismatch", "Unknown format specifier", "Too few format specifiers", "Too many format specifiers", "Scan failed", "Newer CIN version", "Error converting to variant", "Runtime menu error", "Password tampered", "Variant attribute not found", "Incompatible variant data type", "Event data is not available", "Event Store is not present", "Occurrence is not found", "Event Queue is not created", "Event info is not available", "Refnum passed is NULL", "Error retrieving Class GUID", "Error retrieving CoClass GUID", "Error retrieving TypeLib GUID.", "Bad built application magic bytes.", "Specific driver is different from the specific driver associated with the Logical Name.", "There is no session opened to the class driver.", "Max Error", "MAX - Error with config objects", "MAX - Error loading configuration", "MAX - Group not supported"]
        n36 = Format Into String(format string="Software Exception: Unhandled State \"%s\"." ("message"), error in=w80, w78) -> (resulting string=w83:string, error out=w84:errorcluster)  [unwired: 1 in]
        n37 = call <vilib>:"Error Cluster From Error Code.vi"("show call chain? (False)"=TRUE, "error in (no error)"=w84, "error message (\"\")"=w83, "error code (0)"=w82) -> ("error out"=w79:errorcluster)  [unwired: 5 in]
      }
      frame "Initialize" {
        n38 = local read "Averaging samples\n9215"() -> (w96:u32)
        n39 = local read "Degassing rate\n9775"() -> (w95:u32)
        n40 = local read "Data Rate 9215\n(S/s)"() -> (w97:dbl)
        n41 = local read "Data Rate 9775\n(S/s)"() -> (w94:dbl)
        n42 = To Double Precision Float(number=w96) -> (double precision float=w100:dbl)
        n43 = To Double Precision Float(number=w95) -> (double precision float=w93:dbl)
        n44 = Divide(x=w100, y=w97) -> (x/y=w92:dbl)
        n45 = Divide(x=w93, y=w94) -> (x/y=w91:dbl)
        n46 = Max & Min(x=w92, y=w91) -> (min(x,y)=w90:dbl)  [unwired: 1 out]
        n47 = expression code="x*1000"(w90) -> (w99:dbl)
        n48 = To Unsigned Long Integer(number=w99) -> (unsigned 32bit integer=w98:u32)
        n49 = In Range and Coerce(upper limit=u32 20000, x=w98, lower limit=u32 10) -> (coerced(x)=w87:u32)  [unwired: 1 out]
        n50 = Bundle By Name(cluster=w101, "DisplayLoopInterval"=w87) -> (w102:T13)
      }
      frame "Error Handler" {
        n51 = call "General Error Handler - show previous state.vi"("error in (no error)"=w105, "Previous State"=w104, "Loop Select"=enum16{"Event Loop -", "Async Loop -"}."Async Loop -") -> ()  [unwired: 7 in, 2 out]
      }
      frame "CleanUp" {
      }
      frame "Exit" {
        n52 = Flush Queue(queue=w111) -> (queue out=w114:refnum<queue>, error out=w113:errorcluster)  [unwired: 1 in, 1 out]
        n53 = Release Queue(queue=w114, force destroy? (F)=TRUE, error in (no error)=w113) -> ()  [unwired: 3 out]
      }
      frame "", "Idle" {
        n54 = Unbundle By Name(w129) -> ("ProcessingState"=w127:T11)
        n55 = Equal?(x=w127, y=ProcessingState--enum."Running") -> (x = y?=w125:bool)
        n56 = call "FG - DAQ Error Cluster.vi"("action (Get)"=TD_GetSet_ActionSelect--enum."Get") -> ("error out"=w123:errorcluster)  [unwired: 10 in]
        n57 = Unbundle By Name(w123) -> ("source"=w120:string)
        n58 = Unbundle By Name(w123) -> ("status"=w119:bool)
        n59 = call-poly <userlib>:"Data Changed__ogtk.vi"("String"=w120) -> ("Changed"=w122:bool)
        n60 = Compound Arithmetic op=AND(w119, w122) -> (w121:bool)
        n61 = call <userlib>:"Boolean Trigger__ogtk.vi"("Boolean Input"=w119) -> ("Falling Edge"=w118:bool)  [unwired: 1 in, 1 out]
        n62 = case shown="True" w125 {
          tunnel: [w137 w143] -> w131
          tunnel: w130 -> [_ w142]
          tunnel: w128 -> [w135 w140]
          frame False {
            n63 = call <userlib>:"Wait (ms)__ogtk.vi"("error in (no error)"=w135, "milliseconds to wait"=u32 200) -> ("error out"=w137:errorcluster)  [unwired: 8 in, 1 out]
          }
          frame True {
            n64 = call <userlib>:"Wait (ms)__ogtk.vi"("error in (no error)"=w140, "milliseconds to wait"=u32 5) -> ("error out"=w139:errorcluster)  [unwired: 8 in, 1 out]
            n65 = call-poly <vilib>:"Polymorphic - Add States(s) To Queue.vi"("queue in"=w142, "state in"="Action: ReadData", "error in"=w139) -> ("error out"=w143:errorcluster)  [unwired: 9 in, 3 out]
          }
        }
        n66 = local write "DAQError"(w119) -> ()
        n67 = case shown="True" w121 {
          tunnel: w120 -> [_ w134]
          tunnel: w118 -> [w132 _]
          frame False {
            n68 = case shown="True" w132 {
              frame False {
              }
              frame True {
                n69 = property on="DAQError" class="Bool (strict)"("TipStrip"="") -> ()  [unwired: 2 in, 2 out]
              }
            }
          }
          frame True {
            n70 = property on="DAQError" class="Bool (strict)"("TipStrip"=w134) -> ()  [unwired: 2 in, 2 out]
          }
        }
      }
      frame "------ Macro ------" {
      }
      frame "Macro: Initialize" {
        n71 = call-poly <vilib>:"Polymorphic - Add States(s) To Queue.vi"("queue in"=w149, "states in"="Initialize\n/* some state\n/* another state\nIdle", "error in"=w148) -> ("error out"=w147:errorcluster)  [unwired: 10 in, 2 out]
      }
      frame "Macro: Exit" {
        n72 = call-poly <vilib>:"Polymorphic - Add States(s) To Queue.vi"("queue in"=w154, "states in"="/* some state\n/* another state\nCleanUp\nExit", "error in"=w153) -> ("error out"=w152:errorcluster)  [unwired: 10 in, 2 out]
      }
      frame "------ Action ------" {
      }
      frame "Action: ReadData" {
        n73 = Unbundle By Name(w183) -> ("InvWfmsQ-DT"=w172:T17, "DPAuxDataQ"=w164:T18)
        n74 = call "Create Power Data Plots.vi"("error in (no error)"=w176) -> ("error out"=w167:errorcluster, "DUT3 PowerData"=→"DUT3 power data":T20, "DUT2 PowerData"=→"DUT2 power data":T20, "DUT1 PowerData"=→"DUT1 power data":T20, "DUT4 PowerData"=→"DUT4 power data":T20)  [unwired: 6 in]
        n75 = Get Queue Status(queue=w164, error in (no error)=w167) -> (queue out=w173:T18, error out=w166:errorcluster, # elements in queue=→"DP AuxData Size":i32)  [unwired: 1 in, 5 out]
        n76 = Dequeue Element(queue=w173, timeout in ms (-1)=8000, error in (no error)=w166) -> (element=w175:T21[], timed out?=w168:bool, error out=w162:errorcluster)  [unwired: 1 out]
        n77 = Get Queue Status(queue=w172, error in (no error)=w162) -> (queue out=w171:T17, error out=w163:errorcluster, # elements in queue=→"InvWfmsQ DT size":i32)  [unwired: 1 in, 5 out]
        n78 = case shown="False" w168 {
          tunnel: w175 -> [w184 _]
          frame False {
            n79 = for {
              tunnel: w184 -> [w196] mode=indexing
              i -> [w187]
              n80 = Unbundle By Name(w196) -> ("Inv 1 ON?"=w192:bool, "Raw ESR sum"=w190:dbl, "Max ESR"=w189:dbl, "Average scaled ESR sum"=w188:dbl, "Inv 1 over threshold?"=w185:bool, "Inv 1 ESR"=w191:T9)
              n81 = Select(t="RUNNING", s=w192, f="OFF - NO DATA" ("Inverter 1 state:")) -> (s? t:f=w193:string)
              n82 = Bundle("Inverter 1 state:"=w193, "Raw ESR sum"=w190, "Max ESR"=w189, "Average scaled ESR sum"=w188, "Inv 1 over threshold?"=w185) -> (w186:T22)  [unwired: 1 in]
              n83 = case shown="True" w192 {
                tunnel: w187 -> [_ w202]
                tunnel: w191 -> [_ w201]
                frame False {
                }
                frame True {
                  n84 = case shown="3" w202 {
                    tunnel: w201 -> [w203 w204 w205 w206]
                    frame 0, Default {
                      "Equivalent Series Resistance (ESR) 1" <- w203
                    }
                    frame 1 {
                      "Equivalent Series Resistance (ESR) 2" <- w204
                    }
                    frame 2 {
                      "Equivalent Series Resistance (ESR) 3" <- w205
                    }
                    frame 3 {
                      "Equivalent Series Resistance (ESR) 4" <- w206
                    }
                  }
                }
              }
              n85 = case shown="0, Default" w187 {
                tunnel: w186 -> [w197 w198 w199 w200]
                frame 0, Default {
                  "ESR values 1" <- w197
                }
                frame 1 {
                  "ESR values 2" <- w198
                }
                frame 2 {
                  "ESR values 3" <- w199
                }
                frame 3 {
                  "ESR values 4" <- w200
                }
              }
            }
          }
          frame True {
          }
        }
        n86 = Dequeue Element(queue=w171, timeout in ms (-1)=8000, error in (no error)=w163) -> (element=w182:T23, timed out?=w169:bool, error out=w181:errorcluster)  [unwired: 1 out]
        n87 = case shown="False" w169 {
          tunnel: w182 -> [w216 _]
          tunnel: w181 -> [w215 w217]
          tunnel: [w208 w217] -> w177
          frame False {
            n88 = call "Create Graph Plot Arrays.vi"("error in"=w215, "InverterWaveforms"=w216) -> ("error out"=w208:errorcluster, "DUT1 60 Hz V and I"=→"DUT1 I-V":waveform(dbl)[], "Iouts 60Hz"=→"Iout 60Hz":waveform(dbl)[], "DUT4 60 Hz V and I"=→"DUT4 I-V":waveform(dbl)[], "DUT2 60 Hz V and I"=→"DUT2 I-V":waveform(dbl)[], "Iout ripples"=→"Iout ripple":waveform(dbl)[], "DUT3 60 Hz V and I"=→"DUT3 I-V":waveform(dbl)[], "Iin ripples"=→"Iin ripple":waveform(dbl)[])  [unwired: 2 in]
          }
          frame True {
          }
        }
        n89 = call-poly <userlib>:"Filter Error Codes__ogtk.vi"("Error In"=w177, "Error Codes to Filter"=i32[] [1122]) -> ("Error Out"=w160:errorcluster)  [unwired: 7 in, 2 out]
      }
      frame "Action: Wait" {
        n90 = Scan From String(format string="%d", input string=w220, error in=w219, default 1=u32 0) -> (error out=w218:errorcluster, output 1=w224:u32)  [unwired: 1 in, 2 out]
        n91 = call <userlib>:"Wait (ms)__ogtk.vi"("error in (no error)"=w218, "milliseconds to wait"=w224) -> ("error out"=w222:errorcluster)  [unwired: 8 in, 1 out]
      }
      frame "Action: UpdateSMData" {
        n92 = Match Pattern(string=w233, regular expression=":") -> (before substring=w235:string, after substring=w226:string)  [unwired: 1 in, 2 out]
        n93 = case shown="\"ProcessingState\"" w235 {
          tunnel: w232 -> [_ w244]
          tunnel: w231 -> [_ _]
          tunnel: w230 -> [w236 w243]
          tunnel: [w236 w242] -> w229
          tunnel: w228 -> [w237 w241]
          tunnel: [w237 w240] -> w227
          tunnel: w226 -> [_ _]
          frame Default {
            # "#NOTE:\noptionally add error here."
          }
          frame "ProcessingState" {
            n94 = Variant To Data(error in=w241, type=ProcessingState--enum."Idle" ("y"), Variant=w244) -> (data=w238:T11, error out=w240:errorcluster)
            n95 = Bundle By Name(cluster=w243, "ProcessingState"=w238) -> (w242:T13)
          }
        }
      }
    }
  }
  n96 = while {
    shift-right: [w255] -> _
    shift-left: w4 -> [w254]
    shift-right: [w258] -> w3
    shift-left: w6 -> [w253]
    shift-right: [w257] -> _
    shift-left: w9 -> [w259]
    shift-right: [w252] -> _
    shift-left: _ -> [w251]
    tunnel: w8 -> [w249]
    tunnel: w7 -> [w248]
    tunnel: w1 -> [w247]
    stop <- w256 stop-if-true
    n97 = call <vilib>:"Parse State Queue__JKI_lib_State_Machine.vi"("State Queue"=w259, "Error In (no error)"=w253) -> ("Remaining States"=w261:string, "Current State"=w246:string, "Arguments"=w260:string)  [unwired: 11 in]
    n98 = feedback #1(w247) -> (w245:string)
    n99 = feedback-in #1(w246) -> ()
    n100 = case shown="\"UI: Initialize InverterLUT List\"" w246 {
      selector: w246 -> [w263 _ _ _ _ _ _ _ _ _ _ _ _ _ _ _ _ _ _ _ _ _ _ _ _ _ _ _ _ _ _ _ _]
      tunnel: w261 -> [w267 w282 w315 w331 w746 w759 w767 w780 w784 w789 w802 w838 w845 w850 w868 w886 w897 w906 w934 w946 w953 w969 w1021 w1027 w1046 w1051 w1067 w1095 w1127 w1150 w1167 w1179 w1188]
      tunnel: w260 -> [_ _ _ _ _ _ _ _ _ _ _ _ _ _ _ _ _ _ _ _ w948 w964 _ _ _ _ _ _ _ _ _ w1169 _]
      tunnel: w254 -> [w265 w279 w314 w329 w743 w750 w764 w777 w783 w786 w791 w829 w840 w847 w861 w877 w894 w900 w924 w936 w951 w962 w1018 w1024 w1043 w1048 w1063 w1091 w1124 w1147 w1164 w1177 w1185]
      tunnel: [w269 errorcluster {"status"=FALSE, "code"=0, "source"=""} ("error out") w288 w328 w744 w756 w760 w778 w781 w787 w792 w836 w841 w848 w862 w873 w891 w899 w932 w942 w949 w966 w1019 w1025 w1044 w1049 w1065 w1090 w1105 w1137 w1159 w1170 w1180] -> w258
      tunnel: w253 -> [w268 w275 w289 w327 w744 w756 w761 w768 w781 w787 w798 w836 w842 w848 w858 w879 w890 w898 w932 w943 w950 w967 w1019 w1025 w1044 w1049 w1065 w1093 w1104 w1136 w1157 w1171 w1181]
      tunnel: [w266 w281 w323 w330 w745 w758 w766 w780 w784 w788 w801 w837 w844 w849 w867 w885 w896 w905 w933 w945 w952 w968 w1020 w1026 w1045 w1050 w1066 w1094 w1126 w1149 w1166 w1178 w1187] -> w257
      tunnel: [_ _ TRUE _ _ _ _ _ _ _ _ _ _ _ _ _ _ _ _ _ _ _ _ _ _ _ _ _ _ _ _ _ _] -> w256
      tunnel: [w265 w279 w314 w326 w743 w757 w764 w777 w783 w786 w791 w834 w840 w847 w861 w878 w894 w900 w924 w937 w951 w962 w1018 w1024 w1043 w1048 w1063 w1091 w1124 w1147 w1164 w1177 w1185] -> w255
      tunnel: [w262 w277 w321 w324 w742 w747 w765 w779 w782 w785 w800 w833 w839 w846 w866 w884 w895 w904 w925 w944 w947 w963 w1017 w1023 w1039 w1047 w1064 w1092 w1125 w1148 w1165 w1176 w1186] -> w252
      tunnel: w251 -> [w262 w277 w321 w324 w742 w747 w765 _ w782 w785 w800 w833 w839 w846 w866 w884 w895 w904 w925 w944 w947 w963 w1017 w1023 w1039 w1047 w1064 w1092 w1125 w1148 w1165 w1176 w1186]
      tunnel: 200 ("Timeout") -> [_ _ _ w325 _ _ _ _ _ _ _ _ _ _ _ _ _ _ _ _ _ _ _ _ _ _ _ _ _ _ _ _ _]
      tunnel: w249 -> [_ _ _ _ _ _ _ _ _ _ _ _ _ _ _ _ _ _ _ _ _ _ _ w1022 _ _ _ _ _ _ _ _ _]
      tunnel: w248 -> [_ _ _ _ _ _ _ _ _ _ _ _ _ _ _ _ _ _ _ _ _ _ _ _ w1032 _ _ _ _ _ _ _ _]
      tunnel: w245 -> [_ w274 _ _ _ _ _ _ _ _ _ _ _ _ _ _ _ _ _ _ _ _ _ _ _ _ _ _ _ _ _ _ _]
      frame Default {
        w272 = 42 items=["No error", "Argument error", "Memory is full", "Out of zone", "End of file", "File already open", "Generic file I/O error", "File not found", "File permission error", "Disk is full", "Duplicate path", "Too many files open", "System feature not enabled", "Resource file not found", "Cannot add resource", "Resource not found", "Image not found", "Image memory error", "Pen does not exist", "Config type invalid", "Config token not found", "Config parse error", "Config memory error", "Bad external code format", "Bad external code offset", "External code not present", "Null window", "Destroy window error", "Null menu", "Print aborted", "Bad print record", "Print driver error", "Windows error during printing", "Memory error during printing", "Print dialog error", "Generic print error", "Invalid device refnum", "Device not found", "Device parameter error", "Device unit error", "Cannot open device", "Device call aborted", "Generic error", "Cancelled by user", "Object ID too low", "Object ID too high", "Object not in heap", "Unknown heap", "Unknown object (invalid DefProc)", "Unknown object (DefProc not in table)", "Message out of range", "Invalid (null) method", "Unknown message", "Manager call not supported", "Bad address", "Network operation in progress", "Network operation timed out", "Connection is busy", "Network attribute not supported", "Network error", "Address in use", "System out of memory", "Connection aborted", "Connection refused", "Not connected", "Already connected", "Connection closed", "Initialization error (interapplication manager)", "Bad occurrence", "Wait on unbound occurrence handler", "Occurrence queue overflow", "Datalog type conflict", "Unused", "Unrecognized type (interapplication manager)", "Memory corrupt", "Failed to make temporary DLL", "Old CIN version", "Drag socket not found", "Failed to load drop-object", "Failed to register OLE object", "Failed to release OLE object", "Format specifier type mismatch", "Unknown format specifier", "Too few format specifiers", "Too many format specifiers", "Scan failed", "Newer CIN version", "Error converting to variant", "Runtime menu error", "Password tampered", "Variant attribute not found", "Incompatible variant data type", "Event data is not available", "Event Store is not present", "Occurrence is not found", "Event Queue is not created", "Event info is not available", "Refnum passed is NULL", "Error retrieving Class GUID", "Error retrieving CoClass GUID", "Error retrieving TypeLib GUID.", "Bad built application magic bytes.", "Specific driver is different from the specific driver associated with the Logical Name.", "There is no session opened to the class driver.", "Max Error", "MAX - Error with config objects", "MAX - Error loading configuration", "MAX - Group not supported"]
        # "Current State"
        n101 = Format Into String(format string="Software Exception: Unhandled State \"%s\"." ("message"), error in=w268, w263) -> (resulting string=w271:string, error out=w270:errorcluster)  [unwired: 1 in]
        n102 = call <vilib>:"Error Cluster From Error Code.vi"("show call chain? (False)"=TRUE, "error in (no error)"=w270, "error message (\"\")"=w271, "error code (0)"=w272) -> ("error out"=w269:errorcluster)  [unwired: 5 in]
        n103 = call <vilib>:"Add State(s) to Queue__JKI_lib_State_Machine.vi"("State(s) in (\"\")"=w267) -> ("States Out"=w266:string)  [unwired: 14 in]
      }
      frame "Error Handler" {
        n104 = call "General Error Handler - show previous state.vi"("error in (no error)"=w275, "Previous State"=w274, "Loop Select"=enum16{"Event Loop -", "Async Loop -"}."Event Loop -") -> ()  [unwired: 7 in, 2 out]
        n105 = call <vilib>:"Add State(s) to Queue__JKI_lib_State_Machine.vi"("State(s) in Front (\"\")"="/* Post Error States", "State(s) in (\"\")"=w282) -> ("States Out"=w281:string)  [unwired: 13 in]
      }
      frame "Exit" {
        w291 = TRUE  # Overwrite File?
        w304 = 4 ("dimension size")
        n106 = local read "ESR alarm threshhold (%)"() -> (w306:dbl)
        n107 = local read "MinCurrThreshold 1"() -> (w287:dbl)
        n108 = local read "MinCurrThreshold 2"() -> (w286:dbl)
        n109 = local read "MinCurrThreshold 3"() -> (w285:dbl)
        n110 = local read "MinCurrThreshold 4"() -> (w284:dbl)
        n111 = Unbundle By Name(w314) -> ("Core.Current VI Reference"=w316:refnum<vi>)
        n112 = local read "Selected Inverter"() -> (w301:string[])
        n113 = local read "# readings to average"() -> (w308:i32)
        n114 = local read "UseDummyVrms"() -> (w303:bool)
        n115 = local read "Dummy Vrms"() -> (w302:dbl)
        n116 = global read "GBL System.vi" "Config Settings"() -> (w312:T42)
        n117 = local read "ESR scaling"() -> (w310:T7[])
        n118 = local read "Signal scaling"() -> (w309:T3[])
        n119 = Build Array(w287, w286, w285, w284) -> (w283:dbl[])
        n120 = Initialize Array(w306, w304) -> (w305:dbl[])
        n121 = Initialize Array(w308, w304) -> (w307:i32[])
        n122 = local read "Averaging samples\n9215"() -> (w297:u32)
        n123 = Close Reference(reference=w316) -> (error out=w317:errorcluster)  [unwired: 1 in]
        n124 = local read "Data Rate 9775\n(S/s)"() -> (w299:dbl)
        n125 = local read "Data Rate 9215\n(S/s)"() -> (w298:dbl)
        n126 = local read "Degassing rate\n9775"() -> (w296:u32)
        n127 = local read "RIO Device"() -> (w295:T4)
        n128 = Unbundle By Name(w312) -> ("Main Settings"=w311:T14, "DAQ Settings"=w300:T44)
        n129 = Bundle By Name(cluster=w311, "Signal scaling"=w309, "ESR scaling"=w310, "num readings to average"=w307, "ESR alarm threshhold (%)"=w305, "UseDummyVrms"=w303, "Dummy Vrms"=w302, "default Inverter (name)"=w301, "Minimum Current Threshold"=w283) -> (w313:T14)
        n130 = call <userlib>:"Clear All Errors__ogtk.vi"("Error In"=w317) -> ()  [unwired: 3 in, 1 out]
        n131 = call <vilib>:"Add State(s) to Queue__JKI_lib_State_Machine.vi"("State(s) in (\"\")"=w315) -> ("States Out"=w323:string)  [unwired: 14 in]
        n132 = Bundle By Name(cluster=w300, "Initial Measurement settings.Data Rate 9775"=w299, "Initial Measurement settings.Data Rate 9215"=w298, "Initial Measurement settings.Samples RMS 9215"=w297, "Initial Measurement settings.Samples RMS 9775"=w296, "RIO Device"=w295) -> (w294:T44)
        n133 = Bundle By Name(cluster=w312, "Main Settings"=w313, "DAQ Settings"=w294) -> (w290:T42)
        n134 = call "FG - FilePathnames.vi"() -> ("FilePaths out"=w292:T46)  [unwired: 4 in, 1 out]
        n135 = Unbundle By Name(w292) -> ("Config SettingsFile"=w293:path)
        n136 = Current VI's Path() -> (path=w320:path)
        n137 = global write "GBL System.vi" "Config Settings"(w290) -> ()
        n138 = call <vilib>:"show scrollbars v2.vi"("mode (read)"=enum16{"read", "write", "toggle"}."write", "ShowScrollbars?"=TRUE, "vi path"=w320) -> ()  [unwired: 4 in, 2 out]
        n139 = call <vilib>:"Easy Write XML File__JKI EasyXML.vi"("error in (no error)"=w289, "Overwrite File? (false)"=w291, "LabVIEW Data"=w290, "XML File Path"=w293) -> ("error out"=w288:errorcluster)  [unwired: 6 in, 1 out]
      }
      frame "", "Event Structure", "Idle" {
        n140 = event shown="[8] \"Inverter List\": Value Change" {
          selector: w324 -> [_ _ _ _ _ _ _ _ _ _ _ _ _ _ _ _ _ _ _ _ _ _ _ _ _ _ _ _ _ _ _ _ _ _ _]
          dyn-events: _ -> [_ _ _ _ _ _ _ _ _ _ _ _ _ _ _ _ _ _ _ _ _ _ _ _ _ _ _ _ _ _ _ _ _ _ _]
          timeout: w325 -> [_ _ _ _ _ _ _ _ _ _ _ _ _ _ _ _ _ _ _ _ _ _ _ _ _ _ _ _ _ _ _ _ _ _ _]
          tunnel: w331 -> [w337 w343 w350 w357 w363 w391 w400 w405 w420 w425 w429 w436 w448 w466 w485 w494 w525 w546 w554 w563 w570 w584 w597 w602 w614 w618 w626 w634 w642 w654 w708 w716 w723 w737 w741]
          tunnel: [w337 w343 w350 w357 w363 w391 w399 w406 w420 w425 w429 w436 w448 w466 w485 w494 w525 w546 w554 w563 w570 w584 w597 w602 w614 w618 w626 w634 w642 w653 w708 w715 w722 w736 w740] -> w330
          tunnel: w329 -> [w336 w342 w349 w354 w361 w383 w396 w402 w418 w423 w427 w435 w447 w465 w484 w492 w524 w545 w553 w561 w569 w577 w595 w600 w612 w616 w620 w629 w637 w643 w705 w719 w725 w734 w738]
          tunnel: [w334 w340 w345 w353 w362 w386 w398 w407 w419 w424 w428 w432 w445 w457 w482 w493 w523 w543 w551 w560 w566 w583 w596 w601 w609 w617 w625 w633 w641 w651 w703 w720 w726 w735 w739] -> w328
          tunnel: w327 -> [w333 w341 w344 w352 w362 w385 w398 w408 w419 w424 w428 w433 w444 w458 w481 w493 w518 w542 w550 w560 w567 w583 w596 w601 w608 w617 w625 w633 w641 w650 w702 w720 w726 w735 w739]
          tunnel: [w336 w342 w349 w354 w361 w383 w396 w403 w418 w423 w427 w435 w447 w465 w484 w492 w524 w545 w553 w561 w569 w578 w595 w600 w612 w616 w621 w630 w638 w645 w706 w718 w725 w734 w738] -> w326
          event Value Change {
            n141 = event-data() -> ("NewVal"=w332:T1)  [unwired: 1 in]
            n142 = Unbundle By Name(w336) -> ("Dependency.DAQ"=w335:refnum<class "DAQ_Engine.lvclass">)
            n143 = call "CMD SetAcqMode.vi"("error in (no error)"=w333, "Acqusition Mode"=w332, "DAQ_Engine in"=w335) -> ("error out"=w334:errorcluster)  [unwired: 7 in, 1 out]
          }
          event "cRIO Error\nReporting Mode": Value Change {
            n144 = event-data() -> ("NewVal"=w338:i32)  [unwired: 1 in]
            n145 = Unbundle By Name(w342) -> ("Dependency.DAQ"=w339:refnum<class "DAQ_Engine.lvclass">)
            n146 = call "CMD DAQ Error Reporting Mode.vi"("error in (no error)"=w341, "DAQ Error\nReporting Mode"=w338, "DAQ_Engine in"=w339) -> ("error out"=w340:errorcluster)  [unwired: 7 in, 1 out]
          }
          event "DAQEnDis": Value Change {
            # "toggle present state"
            n147 = event-data() -> ()  [unwired: 1 in, 1 out]
            n148 = Unbundle By Name(w349) -> ("DAQEnabled"=w347:bool, "Dependency.DAQ"=w348:refnum<class "DAQ_Engine.lvclass">)
            n149 = Not(x=w347) -> (.not. x?=w346:bool)
            n150 = call "CMD StartStopDAQ.vi"("error in (no error)"=w344, "DAQEnable"=w346, "DAQ_Engine in"=w348) -> ("error out"=w345:errorcluster)  [unwired: 7 in, 1 out]
          }
          event "DAQError": Mouse Down {
            # "Reset system error indicator when mouse down on the indicator"
            n151 = event-data() -> ()  [unwired: 1 in, 8 out]
            n152 = Unbundle By Name(w354) -> ("Dependency.DAQ"=w355:refnum<class "DAQ_Engine.lvclass">)
            n153 = call "Generate Async Cmd Event.vi"("error in (no error)"=w352, "AsyncCmd"=AsynCmd_DAQ_Engine--enum."DAQ.ClearDAQError", "DAQ_Engine in"=w355) -> ("error out"=w353:errorcluster)  [unwired: 7 in, 1 out]
            n154 = local write "DAQError"(FALSE ("SystemError")) -> ()
          }
          event "DataPg_button", "Page2Pg_button", "ConfigPg_button", "SettingsPg_button": Value Change {
            n155 = event-data() -> ("NewVal"=w358:bool, "CtlRef"=w360:refnum<vi>)  [unwired: 1 in]
            n156 = property class="Bool (strict)"(reference=w360) -> ("Label.Text"=w359:string)  [unwired: 1 in, 2 out]
            n157 = case shown="True" w358 {
              selector: w358 -> [_ w368]
              tunnel: w359 -> [_ w370]
              frame False {
              }
              frame True {
                n158 = case shown="\"Page2Pg_button\"" w370 {
                  tunnel: w368 -> [w373 w375 w379 w381]
                  tunnel: [w373 w376 w378 w382] -> w369
                  tunnel: [w372 w375 w378 w382] -> w367
                  tunnel: [w372 w376 w379 w381] -> w366
                  tunnel: [w372 w376 w378 w381] -> w365
                  tunnel: [T2."Data" ("LeftPanelTab") T2."InverterSel" ("LeftPanelTab") T2."Config" ("LeftPanelTab") T2."Settings" ("LeftPanelTab")] -> w364
                  frame "DataPg_button", Default {
                    w372 = FALSE
                  }
                  frame "Page2Pg_button" {
                    w376 = FALSE
                  }
                  frame "ConfigPg_button" {
                    w378 = FALSE
                  }
                  frame "SettingsPg_button" {
                    w382 = FALSE
                  }
                }
                n159 = local write "DataPg_button"(w369) -> ()
                n160 = local write "Page2Pg_button"(w367) -> ()
                n161 = local write "ConfigPg_button"(w366) -> ()
                n162 = local write "SettingsPg_button"(w365) -> ()
                n163 = local write "LeftPanelTab"(w364) -> ()
              }
            }
          }
          event "ESR scaling", "Dummy Vrms", "UseDummyVrms", "Signal scaling": Value Change {
            # "These are used in Process for data processing"
            n164 = event-data() -> ("CtlRef"=w390:refnum<vi>, "NewVal"=w384:variant)  [unwired: 1 in]
            n165 = Unbundle By Name(w383) -> ("Self Reference"=w388:refnum<class "Main.lvclass">)
            n166 = property class="Ctl"(reference=w390, error in=w385) -> (error out=w387:errorcluster, "Label.Text"=w389:string)  [unwired: 1 out]
            n167 = call "Fire UpdateControlValue Event.vi"("error in (no error)"=w387, "vData"=w384, "Control Label"=w389, "Main in"=w388) -> ("error out"=w386:errorcluster)  [unwired: 6 in, 1 out]
          }
          event "Exit": Value Change {
            n168 = event-data() -> ()  [unwired: 1 in, 6 out]
            n169 = call <vilib>:"Three Button Dialog.vi"("Window Title (\"\")"="SYSTEM: Terminate" ("Window Title (\"\")"), "Center Button Text (\"No\")"="", "message"="Terminate Program?") -> ("Which Button?"=w392:T35)  [unwired: 8 in]
            n170 = case shown="Default" w392 {
              tunnel: [_ "Macro: Exit"] -> w397
              frame Default {
              }
              frame "Left Button" {
              }
            }
            n171 = call <vilib>:"Add State(s) to Queue__JKI_lib_State_Machine.vi"("State(s) in Front (\"\")"=w397, "State(s) in (\"\")"=w400) -> ("States Out"=w399:string)  [unwired: 13 in]
          }
          event "Inverter List": Shortcut Menu Selection (User) {
            n172 = event-data() -> ("ItemTag"=w409:string)  [unwired: 1 in, 7 out]
            n173 = case shown="\"View Selected Inverter Param Values\"" w409 {
              tunnel: w408 -> [w411 w414 w417]
              tunnel: [w411 w414 w417] -> w407
              tunnel: [_ "Action: View Inverter Param Values" "Action: Open Inverter LUT DB Editor"] -> w404
              tunnel: w402 -> [w410 w412 w416]
              tunnel: [w410 w412 w416] -> w403
              frame Default {
              }
              frame "View Selected Inverter Param Values" {
              }
              frame "Open Inverter LUT DB Editor" {
              }
            }
            n174 = call <vilib>:"Add State(s) to Queue__JKI_lib_State_Machine.vi"("State(s) in Front (\"\")"=w404, "State(s) in (\"\")"=w405) -> ("States Out"=w406:string)  [unwired: 13 in]
          }
          event "Inverter List": Value Change {
            n175 = event-data() -> ()  [unwired: 1 in, 6 out]
          }
          event "Selected Inverter": Drop {
            n176 = event-data() -> ()  [unwired: 1 in, 1 out]
            n177 = local write "InvSelLED"(FALSE ("InvSelLED")) -> ()
            n178 = event-data("Accepted?"=TRUE) -> ()  [unwired: 1 in, 1 out]
          }
          event "Selected Inverter": Value Change {
            n179 = event-data() -> ()  [unwired: 1 in, 6 out]
            n180 = local write "InvSelLED"(FALSE ("InvSelLED")) -> ()
          }
          event "LogEnDis": Value Change {
            # "toggle present state"
            n181 = event-data() -> ()  [unwired: 1 in, 1 out]
            n182 = Unbundle By Name(w435) -> ("LoggingEnabled"=w434:bool, "Dependency.Log_Engine"=w431:refnum<class "Log_Engine.lvclass">)
            n183 = Not(x=w434) -> (.not. x?=w430:bool)
            n184 = case shown="False" w430 {
              tunnel: w433 -> [w438 w442]
              tunnel: [w437 w441] -> w432
              tunnel: w431 -> [w439 w440]
              frame False {
                n185 = call "CMD StopESRLog.vi"("error in (no error)"=w438, "Log_Engine in"=w439) -> ("error out"=w437:errorcluster)  [unwired: 8 in, 1 out]
              }
              frame True {
                n186 = call "CMD StartESRLog.vi"("error in (no error)"=w442, "Log_Engine in"=w440) -> ("error out"=w441:errorcluster)  [unwired: 8 in, 1 out]
              }
            }
          }
          event "reset averaging": Value Change {
            n187 = event-data() -> ()  [unwired: 1 in, 1 out]
            n188 = Unbundle By Name(w447) -> ("Self Reference"=w446:refnum<class "Main.lvclass">)
            n189 = call "Fire Private Event.vi"("error in (no error)"=w444, "PrivAsync"=PrivateAsynEv_Main--enum."PrivMain.ResetAveraging", "Main in"=w446) -> ("error out"=w445:errorcluster)  [unwired: 7 in, 1 out]
          }
          event "Trigger SelectInverter Event", "SelectInverter": Value Change {
            n190 = event-data() -> ()  [unwired: 1 in, 6 out]
            n191 = Unbundle By Name(w465) -> ("Self Reference"=w464:refnum<class "Main.lvclass">)
            n192 = property class="Main.lvclass"(reference=w464, error in=w458) -> (reference out=w461:refnum<class "Main.lvclass">, error out=w459:errorcluster, "Accessors:InvLUTDict*"=w463:T19, "Accessors:CurrInverter*"=w462:T38[])
            n193 = for {
              tunnel: w463 -> [w474]
              tunnel: w462 -> [w471] mode=indexing
              tunnel: [w468] -> w450 mode=indexing
              tunnel: "Selected Inverter" -> [w467] mode=indexing
              shift-right: [w470] -> w460
              shift-left: w459 -> [w469]
              n194 = call <vilib>:"Get Dynamic CVT Data.vi"("error in (no error)"=w469, "default value (empty variant)"=w471, "DataName"=w467, "dCVT DVR"=w474) -> ("error out"=w472:errorcluster, "value"=w473:variant)  [unwired: 4 in, 2 out]
              n195 = Variant To Data(error in=w472, type=w471, Variant=w473) -> (data=w468:T38, error out=w470:errorcluster)
            }
            n196 = property class="Main.lvclass"(reference=w461, error in=w460, "Accessors:CurrInverter*"=w450) -> (reference out=w455:refnum<class "Main.lvclass">, error out=w453:errorcluster)
            n197 = call "Fire Private Event.vi"("error in (no error)"=w453, "vData"=w450, "PrivAsync"=PrivateAsynEv_Main--enum."PrivMain.CurrInverterUpdated", "Main in"=w455) -> ("error out"=w452:errorcluster, "Main out"=w454:refnum<class "Main.lvclass">)  [unwired: 6 in]
            n198 = call "Generate Async Msg Event.vi"("error in (no error)"=w452, "vData"=w450, "AsyncMsg"=AsynMsg_Main--enum."Main.CurrInverterUpdated", "Main in"=w454) -> ("error out"=w457:errorcluster)  [unwired: 6 in, 1 out]
            n199 = case shown="No Error" w457 {
              frame No Error {
                n200 = local write "InvSelLED"(TRUE ("InvSelLED")) -> ()
              }
              frame Error {
              }
            }
          }
          event "set alarm", "reset alarm": Value Change {
            n201 = event-data() -> ("CtlRef"=w480:refnum<vi>)  [unwired: 1 in]
            n202 = property class="Bool"(reference=w480) -> ("Label.Text"=w479:string)  [unwired: 1 in, 2 out]
            n203 = Equal?(x=w479, y="set alarm") -> (x = y?=w477:bool)
            n204 = Unbundle By Name(w484) -> ("Self Reference"=w483:refnum<class "Main.lvclass">)
            n205 = call "Fire Private Event.vi"("error in (no error)"=w481, "vData"=w477, "PrivAsync"=PrivateAsynEv_Main--enum."PrivMain.SetUnsetAlarm&ESRBLine", "Main in"=w483) -> ("error out"=w482:errorcluster)  [unwired: 6 in, 1 out]
          }
          event "Show_ESR_Data", "Show_TimeSeries_Data", "Show_PowerFactor_Data": Value Change {
            n206 = event-data() -> ("CtlRef"=w491:refnum<vi>)  [unwired: 1 in]
            n207 = property class="Bool"(reference=w491) -> ("Label.Text"=w490:string)  [unwired: 1 in, 2 out]
            n208 = case shown="\"Show_PowerFactor_Data\"" w490 {
              tunnel: [TRUE w500 w503] -> w489
              tunnel: [w497 TRUE w503] -> w488
              tunnel: [w497 w500 TRUE] -> w487
              tunnel: [T6."ESRData" ("MainPanelTab") T6."TimeSeriesData" ("MainPanelTab") T6."PowerFactorData" ("MainPanelTab")] -> w486
              frame "Show_ESR_Data", Default {
                w497 = FALSE
              }
              frame "Show_TimeSeries_Data" {
                w500 = FALSE
              }
              frame "Show_PowerFactor_Data" {
                w503 = FALSE
              }
            }
            n209 = local write "Sel_ESR_Data"(w489) -> ()
            n210 = local write "Sel_TimeSeries_Data"(w488) -> ()
            n211 = local write "Sel_PowerFactor_Data"(w487) -> ()
            n212 = local write "MainPanelTab"(w486) -> ()
          }
          event "StartProcessing": Value Change {
            w521 = T29 {"Inverter ID"=""}  # InverterInfo
            n213 = event-data() -> ()  [unwired: 1 in, 1 out]
            n214 = Unbundle By Name(w524) -> ("Self Reference"=w522:refnum<class "Main.lvclass">, "ProcessingState"=w520:T11)
            n215 = Build Array("MinCurrThreshold 1", "MinCurrThreshold 2", "MinCurrThreshold 3", "MinCurrThreshold 4") -> (w504:dbl[])
            n216 = Not Equal?(x=w520, y=ProcessingState--enum."Running") -> (x != y?=w517:bool)
            n217 = for {
              tunnel: w521 -> [w534]
              tunnel: "Inverter ID" -> [w533]
              tunnel: [w531] -> w515 mode=indexing
              tunnel: [w530] -> w513 mode=indexing
              tunnel: "NumPF RdsToAvg" -> [w529]
              tunnel: "ESR alarm threshhold (%)" -> [w528]
              tunnel: "# readings to average" -> [w527]
              tunnel: w504 -> [w526] mode=indexing
              w532 = T30 {"MinCurrThreshold"=1.5, "NumPF RdsToAvg"=10, "ESR alarm threshhold (%)"=200.0, "# readings to average"=40}  # ProcessInitParams
              n218 = Bundle By Name(cluster=w532, "MinCurrThreshold"=w526, "NumPF RdsToAvg"=w529, "ESR alarm threshhold (%)"=w528, "# readings to average"=w527) -> (w530:T30)
              n219 = Bundle By Name(cluster=w534, "Inverter ID"=w533) -> (w531:T29)
            }
            n220 = Bundle(cluster=T28 {"InverterInfo"=[], "ProcessInitParams"=[]} ("StartProcInitParams"), "InverterInfo"=w515, "ProcessInitParams"=w513) -> (w514:T28)
            n221 = case shown="True" w517 {
              tunnel: w518 -> [w536 w541]
              tunnel: [w537 w540] -> w523
              tunnel: w522 -> [_ w539]
              tunnel: w514 -> [_ w538]
              frame False {
                n222 = call "Dialog Box Timeout v2.vi"("Error In"=w536, "Message"="Data Processing Already Running") -> ("Error Out"=w537:errorcluster)  [unwired: 9 in]
              }
              frame True {
                n223 = call "CMD StartProcessing.vi"("error in (no error)"=w541, "StartProcInitParams"=w538, "Main in"=w539) -> ("error out"=w540:errorcluster)  [unwired: 7 in, 1 out]
              }
            }
          }
          event "StopProcessing": Value Change {
            n224 = event-data() -> ()  [unwired: 1 in, 1 out]
            n225 = Unbundle By Name(w545) -> ("Self Reference"=w544:refnum<class "Main.lvclass">)
            n226 = call "CMD StopProcessing.vi"("error in (no error)"=w542, "Main in"=w544) -> ("error out"=w543:errorcluster)  [unwired: 8 in, 1 out]
          }
          event "StoreESR BLine", "UseSavedESR BLine": Value Change {
            n227 = event-data() -> ()  [unwired: 1 in, 1 out]
            n228 = Unbundle By Name(w553) -> ("Self Reference"=w552:refnum<class "Main.lvclass">)
            n229 = Compound Arithmetic op=OR("StoreESR BLine", "UseSavedESR BLine") -> (w549:bool)
            n230 = case shown="True" w549 {
              tunnel: w552 -> [_ w559]
              tunnel: [w555 w558] -> w551
              tunnel: w550 -> [w555 w557]
              frame False {
              }
              frame True {
                n231 = call "Fire Private Event.vi"("error in (no error)"=w557, "PrivAsync"=PrivateAsynEv_Main--enum."PrivMain.UpdateStoreUseESRBaseline", "Main in"=w559) -> ("error out"=w558:errorcluster)  [unwired: 7 in, 1 out]
              }
            }
          }
          event "SystemError": Mouse Down {
            # "Reset system error indicator when mouse down on the indicator"
            n232 = event-data() -> ()  [unwired: 1 in, 8 out]
            n233 = local write "SystemError"(FALSE ("SystemError")) -> ()
          }
          event "TDMSEnDis": Value Change {
            # "toggle present state"
            n234 = event-data() -> ()  [unwired: 1 in, 1 out]
            n235 = Unbundle By Name(w569) -> ("TDMS Enabled"=w568:bool, "Dependency.Log_Engine"=w565:refnum<class "Log_Engine.lvclass">)
            n236 = Not(x=w568) -> (.not. x?=w564:bool)
            n237 = case shown="False" w564 {
              tunnel: w567 -> [w572 w576]
              tunnel: [w571 w575] -> w566
              tunnel: w565 -> [w573 w574]
              frame False {
                n238 = call "CMD StopLog.vi"("error in (no error)"=w572, "Log_Engine in"=w573) -> ("error out"=w571:errorcluster)  [unwired: 8 in, 1 out]
              }
              frame True {
                n239 = call "CMD StartLog.vi"("error in (no error)"=w576, "Log_Engine in"=w574) -> ("error out"=w575:errorcluster)  [unwired: 8 in, 1 out]
              }
            }
          }
          event "TitleBar", "TitleBar Text", "TitleBar AppVerText": Mouse Down? {
            n240 = event-data() -> ("Button"=w581:u16)  [unwired: 1 in]
            n241 = Unbundle By Name(w577) -> ("Core.Current VI Reference"=w580:refnum<vi>, "MenuBarShown?"=w579:bool)
            n242 = case shown="2" w581 {
              tunnel: w580 -> [_ w587 w592]
              tunnel: w579 -> [_ _ w589]
              tunnel: w577 -> [w585 w586 w591]
              tunnel: [w585 w586 w590] -> w578
              frame 0, Default {
              }
              frame 1 {
                n243 = call "Start Window Drag.vi"("VI Ref (calling VI)"=w587) -> ()  [unwired: 9 in, 2 out]
              }
              frame 2 {
                n244 = Not(x=w589) -> (.not. x?=w588:bool)
                n245 = property class="VI"(reference=w592, "Front Panel.ShowMenuBar"=w588) -> ()  [unwired: 1 in, 2 out]
                n246 = Bundle By Name(cluster=w591, "MenuBarShown?"=w588) -> (w590:T13)
              }
            }
            n247 = event-data("Discard?"=TRUE) -> ()  [unwired: 1 in, 1 out]
          }
          event "toggle MainTabDbgPg": Value Change {
            w594 = FALSE
            n248 = event-data() -> ()  [unwired: 1 in, 3 out]
            n249 = local write "MainPanelTab"(T6."DebugPage" ("MainPanelTab")) -> ()
            n250 = local write "Sel_ESR_Data"(w594) -> ()
            n251 = local write "Sel_TimeSeries_Data"(w594) -> ()
            n252 = local write "Sel_PowerFactor_Data"(w594) -> ()
          }
          event "toggle scrollbars": Value Change {
            n253 = event-data() -> ()  [unwired: 1 in, 3 out]
            n254 = Current VI's Path() -> (path=w599:path)
            n255 = call <vilib>:"show scrollbars v2.vi"("mode (read)"=enum16{"read", "write", "toggle"}."toggle", "vi path"=w599) -> ()  [unwired: 5 in, 2 out]
          }
          event "UpdateDAQSettings": Value Change {
            n256 = event-data() -> ()  [unwired: 1 in, 1 out]
            n257 = Unbundle By Name(w612) -> ("Dependency.DAQ"=w611:refnum<class "DAQ_Engine.lvclass">)
            n258 = global write "GBL System.vi" "RIO Device"("RIO Device") -> ()
            n259 = Bundle By Name(cluster=T5 {"Data Rate 9775"=3.0, "Data Rate 9215"=1200000.0, "Samples RMS 9215"=480000, "Samples RMS 9775"=3} ("MeasSet"), "Data Rate 9775"="Data Rate 9775\n(S/s)", "Data Rate 9215"="Data Rate 9215\n(S/s)", "Samples RMS 9215"="Averaging samples\n9215", "Samples RMS 9775"="Degassing rate\n9775") -> (w610:T5)
            "MeasSet" <- w610
            n260 = call "CMD SetMeasConfig.vi"("error in (no error)"=w608, "MeasSet"=w610, "DAQ_Engine in"=w611) -> ("error out"=w609:errorcluster)  [unwired: 7 in, 1 out]
          }
          event Value Change {
            n261 = event-data() -> ("NewVal"=w615:T4)  [unwired: 1 in]
            n262 = global write "GBL System.vi" "RIO Device"(w615) -> ()
          }
          event User Event {
            n263 = event-data() -> ("NEW State"=w624:T47)  [unwired: 1 in, 6 out]
            n264 = Unbundle By Name(w624) -> ("DAQState"=w623:T31)
            n265 = Equal?(x=w623, y=DAQState--enum."Running" ("DAQState")) -> (x = y?=w619:bool)
            "DAQEnabled" <- w619
            "DAQ Running" <- w619
            n266 = Bundle By Name(cluster=w620, "DAQEnabled"=w619) -> (w621:T13)
          }
          event User Event {
            w628 = LogState--enum."Running"  # LogState
            n267 = event-data() -> ("NEW State"=w632:T49)  [unwired: 1 in, 6 out]
            n268 = Unbundle By Name(w632) -> ("LogState"=w631:T48)
            n269 = Equal?(x=w631, y=w628) -> (x = y?=w627:bool)
            "LogEnabled" <- w627
            n270 = Bundle By Name(cluster=w629, "LoggingEnabled"=w627) -> (w630:T13)
          }
          event User Event {
            w636 = TDMSState--enum."Running"  # TDMSState
            n271 = event-data() -> ("NEW State"=w640:T51)  [unwired: 1 in, 6 out]
            n272 = Unbundle By Name(w640) -> ("TDMSState"=w639:T50)
            n273 = Equal?(x=w639, y=w636) -> (x = y?=w635:bool)
            "TDMSEnabled" <- w635
            n274 = Bundle By Name(cluster=w637, "TDMS Enabled"=w635) -> (w638:T13)
          }
          event User Event {
            n275 = event-data() -> ("CmdMsg"=w648:string, "vData"=w652:variant)  [unwired: 1 in, 1 out]
            n276 = Unbundle By Name(w643) -> ("Self Reference"=w644:refnum<class "Main.lvclass">)
            n277 = call "get async cmd.vi"("error in (no error)"=w650, "Cmd String in"=w648) -> ("error out"=w649:errorcluster, "AsyncCmd"=w647:T52)  [unwired: 8 in]
            n278 = case shown="\"Main.RefreshInverterList\"" w647 {
              tunnel: w652 -> [_ w667 w678 w691]
              tunnel: w649 -> [w660 w666 w677 w690]
              tunnel: [w659 w665 w676 w689] -> w651
              tunnel: [_ "" "" "UI: Initialize InverterLUT List"] -> w646
              tunnel: w643 -> [w655 w663 w674 w688]
              tunnel: [w655 w662 w673 w687] -> w645
              tunnel: w644 -> [_ _ _ _]
              tunnel: w643 -> [_ _ _ _]
              frame Default {
                n279 = call <vilib>:"Build Error Cluster_ModKT .vi"("Prepend String (\"\")"="Invalid Async Cmd" ("Prepend String (\"\")"), "code"=42, "error? (F)"=TRUE, "error in (no error)"=w660) -> ("error out"=w659:errorcluster)  [unwired: 3 in, 1 out]
              }
              frame "Main.StartProcessing" {
                n280 = disable-structure shown="Disabled" {
                  disable-tunnel: w667 -> [w670 _]
                  disable-tunnel: w666 -> [w669 w671]
                  disable-tunnel: [w668 w671] -> w665
                  frame Disabled {
                    n281 = Variant To Data(error in=w669, Variant=w670) -> (error out=w668:errorcluster)  [unwired: 1 in, 1 out]
                  }
                  frame Enabled {
                  }
                }
                n282 = Bundle By Name(cluster=w663, "vData"=variant) -> (w662:T13)
              }
              frame "Main.StopProcessing" {
                n283 = disable-structure shown="Disabled" {
                  disable-tunnel: w678 -> [w681 _]
                  disable-tunnel: w677 -> [w680 w682]
                  disable-tunnel: [w679 w682] -> w676
                  frame Disabled {
                    n284 = Variant To Data(error in=w680, Variant=w681) -> (error out=w679:errorcluster)  [unwired: 1 in, 1 out]
                  }
                  frame Enabled {
                  }
                }
                n285 = Bundle By Name(cluster=w674, "vData"=variant) -> (w673:T13)
              }
              frame "Main.RefreshInverterList" {
                n286 = disable-structure shown="Disabled" {
                  disable-tunnel: w691 -> [w694 _]
                  disable-tunnel: w690 -> [w693 w695]
                  disable-tunnel: [w692 w695] -> w689
                  frame Disabled {
                    n287 = Variant To Data(error in=w693, Variant=w694) -> (error out=w692:errorcluster)  [unwired: 1 in, 1 out]
                  }
                  frame Enabled {
                  }
                }
                n288 = property on="Trigger SelectInverter Event" class="Bool (strict)"() -> ("Value"=w684:bool)  [unwired: 2 in, 2 out]
                n289 = Not(x=w684) -> (.not. x?=w683:bool)
                n290 = property on="Trigger SelectInverter Event" class="Bool (strict)"("Val(Sgnl)"=w683) -> ()  [unwired: 2 in, 2 out]
                n291 = Bundle By Name(cluster=w688, "vData"=variant) -> (w687:T13)
              }
            }
            n292 = call <vilib>:"Add State(s) to Queue__JKI_lib_State_Machine.vi"("State(s) in Front (\"\")"=w646, "State(s) in (\"\")"=w654) -> ("States Out"=w653:string)  [unwired: 13 in]
          }
          event User Event {
            n293 = event-data() -> ("NEW ProcessingState"=w701:T11)  [unwired: 1 in]
            n294 = Unbundle By Name(w705) -> ("SMQ"=w700:refnum<queue>, "Self Reference"=w698:refnum<class "Main.lvclass">)
            n295 = property class="Main.lvclass"(reference=w698) -> ("Accessors:ObjData*"=w697:T53)  [unwired: 1 in, 2 out]
            n296 = call <vilib>:"Add State to Queue with vData.vi"("queue in"=w700, "state in"="Action: UpdateSMData >> ProcessingState", "vData (\"\")"=w701, "error in"=w702) -> ("error out"=w703:errorcluster)  [unwired: 8 in, 3 out]
            n297 = Unbundle By Name(w697) -> ("ESR Chart Ref"=w696:refnum<vi>[])
            n298 = for {
              tunnel: w696 -> [w709] mode=indexing
              n299 = property on="Property Node" class="WFChart (strict)"(reference=w709, "YScale.FormatString"="%#_g" ("Y Scale.Format String"), "YScale.Minimum"=0.0 ("Y Scale.Range:Minimum"), "YScale.Maximum"=0.1 ("Y Scale.Range:Maximum"), "History Data"=T32 []) -> ()  [unwired: 1 in, 2 out]
            }
            n300 = Equal?(x=w701, y=ProcessingState--enum."Running") -> (x = y?=→"Processing":bool)
            n301 = Bundle By Name(cluster=w705, "ProcessingState"=w701) -> (w706:T13)
          }
          event User Event {
            n302 = event-data() -> ("notifier out"=w717:refnum<notifier>)  [unwired: 1 in]
            n303 = Bundle By Name(cluster=w719, "process sync"=w717) -> (w718:T13)
            n304 = call <vilib>:"Add State(s) to Queue__JKI_lib_State_Machine.vi"("State(s) in Front (\"\")"="Macro: Exit", "State(s) in (\"\")"=w716) -> ("States Out"=w715:string)  [unwired: 13 in]
          }
          event Menu Selection (User) {
            n305 = event-data() -> ("ItemTag"=w724:string)  [unwired: 1 in, 2 out]
            n306 = case shown="\"Launch ESR Gain & Offset Explorer\"" w724 {
              tunnel: ["" "Macro: Exit" "UI: Launch TDMS Viewer" "UI: Show About Dialog" "UI: Launch ESR Gain&Offset Explorer"] -> w721
              frame Default {
              }
              frame "Exit" {
              }
              frame "TDMS File Viewer" {
              }
              frame "About" {
              }
              frame "Launch ESR Gain & Offset Explorer" {
              }
            }
            n307 = call <vilib>:"Add State(s) to Queue__JKI_lib_State_Machine.vi"("State(s) in Front (\"\")"=w721, "State(s) in (\"\")"=w723) -> ("States Out"=w722:string)  [unwired: 13 in]
          }
          event Panel Close? {
            n308 = event-data() -> ()  [unwired: 1 in, 1 out]
            n309 = call <vilib>:"Add State(s) to Queue__JKI_lib_State_Machine.vi"("State(s) in Front (\"\")"="Macro: Exit", "State(s) in (\"\")"=w737) -> ("States Out"=w736:string)  [unwired: 13 in]
            n310 = event-data("Discard?"=TRUE) -> ()  [unwired: 1 in, 1 out]
          }
          event Timeout {
            n311 = event-data() -> ()  [unwired: 1 in, 1 out]
            n312 = call <vilib>:"Add State(s) to Queue__JKI_lib_State_Machine.vi"("State(s) in (\"\")"=w741) -> ("States Out"=w740:string)  [unwired: 14 in]
          }
        }
      }
      frame "---------- Core ----------" {
        n313 = call <vilib>:"Add State(s) to Queue__JKI_lib_State_Machine.vi"("State(s) in (\"\")"=w746) -> ("States Out"=w745:string)  [unwired: 14 in]
      }
      frame "Initialize Core Data" {
        # "originally closed?"
        # "exe?"
        n314 = property class="VI"() -> ("Front Panel.Open"=w755:bool)  [unwired: 2 in, 2 out]
        n315 = property class="App"() -> ("App.Kind"=w754:T33)  [unwired: 2 in, 2 out]
        n316 = control-ref of="Current VI Reference"() -> (w748:refnum<vi>)
        n317 = Not(x=w755) -> (.not. x?=w752:bool)
        n318 = Equal?(x=w754, y=T33."Run Time System" ("Application:Kind")) -> (x = y?=w751:bool)
        n319 = Or(x=w752, y=w751) -> (x .or. y?=w749:bool)
        n320 = Bundle By Name(cluster=w750, "Core.Current VI Reference"=w748, "Core.Close Panel on Exit?"=w749) -> (w757:T13)
        n321 = call <vilib>:"Add State(s) to Queue__JKI_lib_State_Machine.vi"("State(s) in (\"\")"=w759) -> ("States Out"=w758:string)  [unwired: 14 in]
      }
      frame "Process Sync" {
        n322 = Unbundle By Name(w764) -> ("process sync"=w763:refnum<notifier>)
        n323 = Send Notification(notification=TRUE, notifier=w763, error in (no error)=w761) -> (error out=w760:errorcluster)  [unwired: 1 out]
        n324 = call <vilib>:"Add State(s) to Queue__JKI_lib_State_Machine.vi"("State(s) in (\"\")"=w767) -> ("States Out"=w766:string)  [unwired: 14 in]
      }
      frame "DE_Register" {
        n325 = Unbundle By Name(w777) -> ("Public Events"=w776:T16, "Dependency.DAQ"=w775:refnum<class "DAQ_Engine.lvclass">, "Dependency.Log_Engine"=w773:refnum<class "Log_Engine.lvclass">)
        n326 = property class="DAQ_Engine.lvclass"(reference=w775, error in=w768) -> (error out=w770:errorcluster, "Accessors:PublicEvents*"=w774:T60)  [unwired: 1 out]
        n327 = property class="Log_Engine.lvclass"(reference=w773, error in=w768) -> (error out=w771:errorcluster, "Accessors:PublicEvents*"=w772:T61)  [unwired: 1 out]
        n328 = Merge Errors(w770, w771) -> (w769:errorcluster)
        n329 = register-events(error in=w769, w776, w774, w772) -> (reference out=w779:refnum<event-registration>, error out=w778:errorcluster)  [unwired: 1 in]
      }
      frame "DE_Unregister" {
        n330 = Unregister For Events(event registration refnum=w782, error in=w781) -> ()  [unwired: 1 out]
      }
      frame "---------- Data ----------" {
        n331 = call <vilib>:"Add State(s) to Queue__JKI_lib_State_Machine.vi"("State(s) in (\"\")"=w789) -> ("States Out"=w788:string)  [unwired: 14 in]
      }
      frame "Data: CreateCtrlRefs" {
        (unwired) "CtrlLabel-IOName Config - TS.xml" ("name or relative path")
        # "#TODO: finish implementation"
        n332 = Unbundle By Name(w791) -> ()  [unwired: 1 out]
        n333 = Unbundle By Name(w791) -> ("Application"=w790:refnum<class "Application.lvclass">)
        n334 = call <userlib>:"Wait (ms)__ogtk.vi"("error in (no error)"=w798, "milliseconds to wait"=u32 4000) -> ("error out"=w793:errorcluster)  [unwired: 8 in, 1 out]
        n335 = call "FG - App Class Ref.vi"("Application in"=w790, "error in (no error)"=w793, "action (Get)"=TD_GetSet_ActionSelect--enum."Set") -> ("Application out"=w795:refnum<class "Application.lvclass">, "error out"=w794:errorcluster)  [unwired: 6 in]
        n336 = call "Generate Async Msg Event.vi"("error in (no error)"=w794, "AsyncMsg"=AsynMsg_Application--enum."Application.AppClassReference", "Application in"=w795) -> ("error out"=w792:errorcluster)  [unwired: 7 in, 1 out]
        n337 = call <vilib>:"Add State(s) to Queue__JKI_lib_State_Machine.vi"("State(s) in (\"\")"=w802) -> ("States Out"=w801:string)  [unwired: 14 in]
      }
      frame "Data: Initialize" {
        w820 = FALSE ("DAQ Running")
        w835 = T62 {"Current VI Reference"=refnum, "Close Panel on Exit?"=FALSE}  # Core
        # "#TODO: add more items for\ninitialization here."
        n338 = Unbundle By Name(w829) -> ("DAQEnabled"=w828:bool, "LoggingEnabled"=w827:bool, "TDMS Enabled"=w826:bool, "Settings.Signal scaling"=w825:T3[], "Settings.ESR scaling"=w818:T7[], "Settings.num readings to average"=w824:i32[], "Settings.ESR alarm threshhold (%)"=w823:i32[], "Settings.UseDummyVrms"=w822:bool, "Settings.Dummy Vrms"=w821:dbl, "Dependency.DAQ"=w817:refnum<class "DAQ_Engine.lvclass">, "Settings.Minimum Current Threshold"=w807:dbl[])  [unwired: 1 out]
        n339 = property class="DAQ_Engine.lvclass"(reference=w817) -> ("Accessors:MeasSettings*"=w816:T5, "Accessors:Settings*"=w809:T44)  [unwired: 1 in, 2 out]
        n340 = Unbundle By Name(w829) -> ("StatusMsg Ref"=w831:refnum<vi>)
        n341 = Index Array(array=w823) -> (element=w810:i32)  [unwired: 1 in]
        n342 = Unbundle By Name(w816) -> ("Data Rate 9775"=w815:dbl, "Data Rate 9215"=w814:dbl, "Samples RMS 9215"=w813:u32, "Samples RMS 9775"=w812:u32)
        n343 = Unbundle By Name(w809) -> ("RIO Device"=w808:string)
        n344 = Index Array(array=w824) -> (element=w811:i32)  [unwired: 1 in]
        n345 = call <vilib>:"format status message v2.vi"("status msg"="Running Main UI", "Str Refnum"=w831) -> ()  [unwired: 5 in, 5 out]
        n346 = local write "Signal scaling"(w825) -> ()
        n347 = local write "ESR scaling"(w818) -> ()
        n348 = local write "# readings to average"(w811) -> ()
        n349 = local write "ESR alarm threshhold (%)"(w810) -> ()
        n350 = local write "UseDummyVrms"(w822) -> ()
        n351 = local write "DAQEnabled"(w828) -> ()
        n352 = local write "LogEnabled"(w827) -> ()
        n353 = local write "TDMSEnabled"(w826) -> ()
        n354 = local write "Dummy Vrms"(w821) -> ()
        n355 = local write "Averaging samples\n9215"(w813) -> ()
        n356 = local write "Data Rate 9775\n(S/s)"(w815) -> ()
        n357 = local write "Data Rate 9215\n(S/s)"(w814) -> ()
        n358 = local write "Degassing rate\n9775"(w812) -> ()
        n359 = local write "RIO Device"(w808) -> ()
        n360 = Current VI's Menubar() -> (w832:refnum<k9>)
        n361 = local write "DAQ Running"(w820) -> ()
        n362 = local write "Processing"(w820) -> ()
        n363 = local write "Inverter ID"("") -> ()
        n364 = Bundle By Name(cluster=w829, "Core"=w835, "MenuRef"=w832) -> (w834:T13)
        n365 = Index Array(array=w807) -> (element #1=w806:dbl, element #2=w805:dbl, element #3=w804:dbl, element #4=w803:dbl)  [unwired: 4 in]
        n366 = local write "MinCurrThreshold 1"(w806) -> ()
        n367 = local write "MinCurrThreshold 2"(w805) -> ()
        n368 = local write "MinCurrThreshold 3"(w804) -> ()
        n369 = local write "MinCurrThreshold 4"(w803) -> ()
        n370 = call <vilib>:"Add State(s) to Queue__JKI_lib_State_Machine.vi"("State(s) in (\"\")"=w838) -> ("States Out"=w837:string)  [unwired: 14 in]
      }
      frame "Data: Cleanup" {
        n371 = Unbundle By Name(w840) -> ("Core.Current VI Reference"=w843:refnum<vi>)
        n372 = Close Reference(reference=w843, error in (no error)=w842) -> (error out=w841:errorcluster)
        n373 = call <vilib>:"Add State(s) to Queue__JKI_lib_State_Machine.vi"("State(s) in (\"\")"=w845) -> ("States Out"=w844:string)  [unwired: 14 in]
      }
      frame "---------- UI ----------" {
        n374 = call <vilib>:"Add State(s) to Queue__JKI_lib_State_Machine.vi"("State(s) in (\"\")"=w850) -> ("States Out"=w849:string)  [unwired: 14 in]
      }
      frame "UI: Launch ESR Gain&Offset Explorer" {
        n375 = control-ref of="ESR scaling"() -> (w859:refnum<vi>)
        n376 = vi-ref "Control UI - Gain and Offset Exploration.vi"() -> (w856:refnum<vi>)
        n377 = case shown="\"DUT1\", Default" "Tab Control" {
          tunnel: [0 1 2 3] -> w851
          frame "DUT1", Default {
          }
          frame "DUT2" {
          }
          frame "DUT3" {
          }
          frame "DUT4" {
          }
        }
        n378 = Unbundle By Name(w861) -> ("Self Reference"=w860:refnum<class "Main.lvclass">)
        n379 = property class="VI"(reference=w856) -> ("Path"=w855:path)  [unwired: 1 in, 2 out]
        n380 = Open VI Reference(type specifier VI Refnum (for type only)=refnum<vi> refnum, vi path=w855, options=128, error in (no error)=w858) -> (vi reference=w853:refnum<vi>, error out=w857:errorcluster)  [unwired: 2 in]
        n381 = call-by-ref "Start Asynchronous Call"(reference=w853, error in=w857, "index"=w851, "ESR scaling ref"=w859, "Main Ref"=w860) -> (reference out=w864:refnum<vi>, error out=w863:errorcluster)  [unwired: 9 in]
        n382 = Close Reference(reference=w864, error in (no error)=w863) -> (error out=w862:errorcluster)
        n383 = call <vilib>:"Add State(s) to Queue__JKI_lib_State_Machine.vi"("State(s) in (\"\")"=w868) -> ("States Out"=w867:string)  [unwired: 14 in]
      }
      frame "UI: Initialize InverterLUT List" {
        n384 = Unbundle By Name(w877) -> ("Self Reference"=w883:refnum<class "Main.lvclass">)
        n385 = property class="Main.lvclass"(reference=w883, error in=w879) -> (error out=w880:errorcluster, "Accessors:InvLUTDict*"=w882:T19, "Accessors:CurrInverter*"=w881:T38[])  [unwired: 1 out]
        n386 = for {
          tunnel: w881 -> [w888] mode=indexing
          tunnel: [w887] -> w876 mode=indexing
          n387 = Unbundle By Name(w888) -> ("name"=w887:string)
        }
        n388 = local write "Selected Inverter"(w876) -> ()
        n389 = call <vilib>:"Get ALL Dynamic CVT Data.vi"("error in (no error)"=w880, "dCVT DVR"=w882) -> ("error out"=w873:errorcluster, "NameArray"=w875:string[], "dCVT DVR out"=w874:T19)  [unwired: 6 in, 1 out]
        n390 = case shown="No Error" w873 {
          frame No Error {
            n391 = local write "InvSelLED"(TRUE ("InvSelLED")) -> ()
          }
          frame Error {
          }
        }
        n392 = Bundle By Name(cluster=w877, "InverterLUT Dict"=w874, "InverterNames[]"=w875) -> (w878:T13)
        n393 = property on="Inverter List" class="LstBox (strict)"("Item Names"=w875) -> ()  [unwired: 2 in, 2 out]
        n394 = call <vilib>:"Add State(s) to Queue__JKI_lib_State_Machine.vi"("State(s) in (\"\")"=w886) -> ("States Out"=w885:string)  [unwired: 14 in]
      }
      frame "UI: Show About Dialog" {
        n395 = Unbundle By Name(w894) -> ("Core.Current VI Reference"=w893:refnum<vi>)
        n396 = global read "GBL System.vi" "AppVersion"() -> (w892:string)
        n397 = call "Call About Dialog.vi"("error in (no error)"=w890, "AppVer"=w892, "Main UI Ref"=w893) -> ("error out"=w891:errorcluster)  [unwired: 8 in]
        n398 = call <vilib>:"Add State(s) to Queue__JKI_lib_State_Machine.vi"("State(s) in (\"\")"=w897) -> ("States Out"=w896:string)  [unwired: 14 in]
      }
      frame "UI: Launch TDMS Viewer" {
        n399 = Unbundle By Name(w900) -> ("TDMS Enabled"=w901:bool)
        n400 = case shown="True" w901 {
          tunnel: "Do Not Open TDMS File While System is Writing to File." ("message") -> [_ w923]
          tunnel: [T35."Left Button" ("Which Button?") w919] -> w903
          frame False {
          }
          frame True {
            n401 = call <vilib>:"Three Button Dialog.vi"("Window Title (\"\")"="CAUTION" ("Window Title (\"\")"), "Center Button Text (\"No\")"="", "Left Button Text (\"Yes\")"="OK", "message"=w923) -> ("Which Button?"=w919:T35)  [unwired: 7 in]
          }
        }
        n402 = case shown="Default" w903 {
          tunnel: w898 -> [w916 w917]
          tunnel: [w915 w917] -> w899
          frame Default {
            n403 = vi-ref "Launch TDMS File Viewer.vi"() -> (w907:refnum<vi>)
            n404 = property class="VI"(reference=w907) -> ("Path"=w908:path)  [unwired: 1 in, 2 out]
            n405 = Open VI Reference(type specifier VI Refnum (for type only)=refnum<vi> refnum, vi path=w908, options=128, error in (no error)=w916) -> (vi reference=w914:refnum<vi>, error out=w911:errorcluster)  [unwired: 2 in]
            n406 = call-by-ref "Start Asynchronous Call"(reference=w914, error in=w911) -> (reference out=w910:refnum<vi>, error out=w909:errorcluster)  [unwired: 12 in]
            n407 = Close Reference(reference=w910, error in (no error)=w909) -> (error out=w915:errorcluster)
          }
          frame "Right Button" {
          }
        }
        n408 = call <vilib>:"Add State(s) to Queue__JKI_lib_State_Machine.vi"("State(s) in (\"\")"=w906) -> ("States Out"=w905:string)  [unwired: 14 in]
      }
      frame "UI: Initialize2" {
        w927 = FALSE
        w930 = FALSE
        n409 = Unbundle By Name(w924) -> ()  [unwired: 1 out]
        n410 = local write "MainPanelTab"(T6."ESRData" ("MainPanelTab")) -> ()
        n411 = local write "DataPg_button"(w930) -> ()
        n412 = local write "Page2Pg_button"(w930) -> ()
        n413 = local write "ConfigPg_button"(w930) -> ()
        n414 = local write "SettingsPg_button"(TRUE) -> ()
        n415 = local write "LeftPanelTab"(T2."Settings" ("LeftPanelTab")) -> ()
        n416 = local write "Sel_ESR_Data"(TRUE) -> ()
        n417 = local write "Sel_TimeSeries_Data"(w927) -> ()
        n418 = local write "Sel_PowerFactor_Data"(w927) -> ()
        n419 = call <vilib>:"Add State(s) to Queue__JKI_lib_State_Machine.vi"("State(s) in (\"\")"=w934) -> ("States Out"=w933:string)  [unwired: 14 in]
      }
      frame "UI: Initialize" {
        w935 = TRUE
        # "#TODO: add Remote error handling menu items"
        n420 = Unbundle By Name(w936) -> ("Core.Current VI Reference"=w941:refnum<vi>)
        n421 = call <userlib>:"Fit VI window to Largest Dec__ogtk.vi"("error in (no error)"=w943, "VI Ref (calling VI)"=w941) -> ("error out"=w942:errorcluster, "dup VI Ref"=w940:refnum<vi>)  [unwired: 4 in]
        n422 = global read "GBL System.vi" "AppVersion"() -> (w939:string)
        n423 = local write "TitleBar AppVerText"(w939) -> ()
        n424 = property class="VI"(reference=w940, "Front Panel.Title"=w939) -> (reference out=w938:refnum<vi>)  [unwired: 1 in, 1 out]
        n425 = Bundle By Name(cluster=w936, "MenuBarShown?"=w935) -> (w937:T13)
        n426 = property class="VI"(reference=w938, "Front Panel.ShowMenuBar"=w935) -> ()  [unwired: 1 in, 2 out]
        n427 = call <vilib>:"Add State(s) to Queue__JKI_lib_State_Machine.vi"("State(s) in (\"\")"=w946) -> ("States Out"=w945:string)  [unwired: 14 in]
      }
      frame "UI: Cursor Set" {
        # "Argument"
        n428 = case shown="\"Idle\", Default" w948 {
          tunnel: w950 -> [w955 w957]
          tunnel: [w954 w956] -> w949
          frame "Idle", Default {
            n429 = call <vilib>:"Unset Busy.vi"("error in (no error)"=w955) -> ("error out"=w954:errorcluster)  [unwired: 10 in]
          }
          frame "Busy" {
            n430 = call <vilib>:"Set Busy.vi"("error in (no error)"=w957) -> ("error out"=w956:errorcluster)  [unwired: 9 in, 1 out]
          }
        }
        n431 = call <vilib>:"Add State(s) to Queue__JKI_lib_State_Machine.vi"("State(s) in (\"\")"=w953) -> ("States Out"=w952:string)  [unwired: 14 in]
      }
      frame "UI: Front Panel State" {
        # "Argument"
        n432 = Unbundle By Name(w962) -> ("Core.Current VI Reference"=w965:refnum<vi>)
        n433 = Unbundle By Name(w962) -> ("Splash VI Ref"=w961:refnum<vi>, "Splash StatusRef"=w958:refnum<vi>, "StatusMsg Ref"=w959:refnum<vi>)
        n434 = case shown="\"Open\", Default" w964 {
          tunnel: w967 -> [w973 w992]
          tunnel: [w975 w984] -> w966
          tunnel: w965 -> [w974 w990]
          tunnel: w961 -> [_ w987]
          tunnel: "Quitting  IHS\nPlease Wait . . ." ("FP Msg") -> [_ w986]
          tunnel: w958 -> [_ w982]
          tunnel: w959 -> [_ w983]
          frame "Open", Default {
            n435 = property class="VI"(reference=w974, error in=w973) -> (reference out=w971:refnum<vi>, error out=w972:errorcluster, "Front Panel.Open"=w970:bool)
            n436 = case shown="False" w970 {
              tunnel: [w978 w981] -> w975
              tunnel: w972 -> [w977 w981]
              tunnel: w971 -> [w976 _]
              frame False {
                n437 = invoke class="VI" method="FP.Open"(reference=w976, error in=w977, "Activate"=TRUE, "State"=T36."Standard") -> (error out=w978:errorcluster)  [unwired: 1 in, 4 out]
              }
              frame True {
              }
            }
          }
          frame "Close" {
            n438 = property class="VI"(reference=w990, error in=w992) -> (reference out=w989:refnum<vi>, error out=w991:errorcluster, "Front Panel.Open"=w988:bool)
            n439 = case shown="True" w988 {
              tunnel: [w1013 w1016] -> w985
              tunnel: w991 -> [w1013 w1015]
              tunnel: w989 -> [_ w1014]
              frame False {
              }
              frame True {
                n440 = invoke class="VI" method="FP.Close"(reference=w1014, error in=w1015) -> (error out=w1016:errorcluster)  [unwired: 1 in, 2 out]
              }
            }
            n441 = disable-structure shown="Disabled" {
              disable-tunnel: w987 -> [w1008 _]
              disable-tunnel: w986 -> [w1006 _]
              disable-tunnel: w985 -> [w1004 w1012]
              disable-tunnel: [w1003 w1012] -> w984
              disable-tunnel: w983 -> [w994 _]
              disable-tunnel: w982 -> [w993 _]
              frame Disabled {
                n442 = property class="Str"(reference=w994) -> (error out=w995:errorcluster, "Value"=w999:string)  [unwired: 1 in, 1 out]
                n443 = call "FG - StatusStrRef.vi"("StatusStr Ref in"=w993, "error in (no error)"=w995, "action (Get)"=TD_GetSet_ActionSelect--enum."Set") -> ("StatusStr Ref out"=w997:refnum<vi>, "error out"=w996:errorcluster)  [unwired: 6 in]
                n444 = call <userlib>:"Set Control Value {Variant}__ogtk.vi"("error in (no error)"=w1004, "Control Name (\"\": use variant name)"="FP Msg", "Value"=w1006, "VI Refnum"=w1008) -> ("error out"=w1005:errorcluster, "VI Refnum dup"=w1009:refnum<vi>)  [unwired: 6 in]
                n445 = property class="Str"(reference=w997, error in=w996, "Value"=w999) -> (reference out=w1000:refnum<vi>, error out=w1001:errorcluster)
                n446 = property class="VI"(reference=w1009, error in=w1005, "FP.Behavior"=T37."Modal" ("Front Panel Window:Behavior"), "FP.State"=T36."Standard" ("Front Panel Window:State")) -> (error out=w1003:errorcluster)  [unwired: 1 out]
                n447 = property class="Str"(reference=w1000, error in=w1001, "Text.Scroll Position"=u32 999999999) -> ()  [unwired: 2 out]
              }
              frame Enabled {
              }
            }
          }
        }
        n448 = call <vilib>:"Add State(s) to Queue__JKI_lib_State_Machine.vi"("State(s) in (\"\")"=w969) -> ("States Out"=w968:string)  [unwired: 14 in]
      }
      frame "---------- Macro ----------" {
        n449 = call <vilib>:"Add State(s) to Queue__JKI_lib_State_Machine.vi"("State(s) in (\"\")"=w1021) -> ("States Out"=w1020:string)  [unwired: 14 in]
      }
      frame "Macro: Initialize" {
        n450 = call <vilib>:"Add State(s) to Queue__JKI_lib_State_Machine.vi"("State(s) in Front (\"\")"=w1022, "State(s) in (\"\")"=w1027) -> ("States Out"=w1026:string)  [unwired: 13 in]
      }
      frame "Macro: Exit" {
        n451 = Unbundle By Name(w1043) -> ("Core.Close Panel on Exit?"=w1042:bool, "LoggingEnabled"=w1033:bool, "TDMS Enabled"=w1035:bool, "DAQEnabled"=w1034:bool)
        n452 = Compound Arithmetic op=OR(w1033, w1035, w1034) -> (w1031:bool)
        n453 = Select(t="Action: Stop Daq & Logging", s=w1031, f="") -> (s? t:f=w1028:string)
        n454 = call <vilib>:"Add State(s) to Queue__JKI_lib_State_Machine.vi"("State(s) in Front (\"\")"=w1028, "State(s) in (\"\")"=w1032) -> ("States Out"=w1036:string)  [unwired: 13 in]
        n455 = Select(t="UI: Front Panel State >> Close", s=w1042, f="") -> (s? t:f=w1038:string)
        n456 = Format Into String(format string=w1036, w1038) -> (resulting string=w1037:string)  [unwired: 2 in, 1 out]
        n457 = call <vilib>:"Add State(s) to Queue__JKI_lib_State_Machine.vi"("State(s) in Front (\"\")"=w1037, "State(s) in (\"\")"=w1046) -> ("States Out"=w1045:string)  [unwired: 13 in]
      }
      frame "---------- Action ----------" {
        n458 = call <vilib>:"Add State(s) to Queue__JKI_lib_State_Machine.vi"("State(s) in (\"\")"=w1051) -> ("States Out"=w1050:string)  [unwired: 14 in]
      }
      frame "Action: Open Inverter LUT DB Editor" {
        n459 = Unbundle By Name(w1063) -> ("Self Reference"=w1054:refnum<class "Main.lvclass">, "Core.Current VI Reference"=w1052:refnum<vi>)
        n460 = vi-ref "Inverter LUT UI.vi"() -> (w1058:refnum<vi>)
        n461 = property class="VI (strict)"(reference=w1058) -> (reference out=w1055:refnum<vi>, "Path"=w1057:path)  [unwired: 1 in, 1 out]
        n462 = Open VI Reference(type specifier VI Refnum (for type only)=w1055, vi path=w1057, options=128) -> (vi reference=w1056:refnum<vi>, error out=w1060:errorcluster)  [unwired: 3 in]
        n463 = call-by-ref "Start Asynchronous Call"(reference=w1056, error in=w1060, "Caller VI Refnum (Callee's Caller)"=w1052, "Main in"=w1054) -> (reference out=w1053:refnum<vi>, error out=w1061:errorcluster)  [unwired: 9 in, 1 out]
        n464 = Close Reference(reference=w1053, error in (no error)=w1061) -> (error out=w1062:errorcluster)
        n465 = call <userlib>:"Clear All Errors__ogtk.vi"("Error In"=w1062) -> ()  [unwired: 3 in, 1 out]
        n466 = call <vilib>:"Add State(s) to Queue__JKI_lib_State_Machine.vi"("State(s) in (\"\")"=w1067) -> ("States Out"=w1066:string)  [unwired: 14 in]
      }
      frame "Action: View Inverter Param Values" {
        n467 = Unbundle By Name(w1091) -> ("Core.Current VI Reference"=w1079:refnum<vi>)
        n468 = local read "Inverter List"() -> (w1069:i32[])
        n469 = Unbundle By Name(w1091) -> ("Self Reference"=w1080:refnum<class "Main.lvclass">)
        n470 = property on="Inverter List" class="LstBox (strict)"() -> ("Item Names"=w1078:string[])  [unwired: 2 in, 2 out]
        n471 = Index Array(array=w1069) -> (element=w1068:i32)  [unwired: 1 in]
        n472 = property class="Main.lvclass"(reference=w1080) -> (error out=w1075:errorcluster, "Accessors:InvLUTDict*"=w1077:T19)  [unwired: 1 in, 1 out]
        n473 = Index Array(array=w1078, index=w1068) -> (element=w1076:string)
        n474 = vi-ref "View Selected Inverter Parameter Values.vi"() -> (w1081:refnum<vi>)
        n475 = property class="VI (strict)"(reference=w1081) -> (reference out=w1083:refnum<vi>, "Path"=w1085:path)  [unwired: 1 in, 1 out]
        n476 = Open VI Reference(type specifier VI Refnum (for type only)=w1083, vi path=w1085, options=128) -> (vi reference=w1084:refnum<vi>, error out=w1087:errorcluster)  [unwired: 3 in]
        n477 = call <vilib>:"Get Dynamic CVT Data.vi"("error in (no error)"=w1075, "DataName"=w1076, "dCVT DVR"=w1077) -> ("error out"=w1073:errorcluster, "value"=w1074:variant)  [unwired: 5 in, 2 out]
        n478 = Variant To Data(error in=w1073, type=T38 {"name"="", "last updated"=timestamp(0 s since 1904-01-01), "type"="", "inverter Info"={"manufacturer"="", "model"="", "product"="", "serial"="", "power class"="", "year manf"=""}, "gain range"={"gain max"=0.0, "gain min"=0.0, "gain increment"=0.0}, "offset range"={"offset max"=0.0, "offset min"=0.0, "offset increment"=0.0}, "gain actual"=0.0, "offset actual"=0.0, "power level"=0.0, "minimum current"=0.0, "resistance single phase"=0.0, "resistance 3 phase"=0.0, "set flag"=0} ("Inverter v2"), Variant=w1074) -> (data=w1072:T38, error out=w1071:errorcluster)
        n479 = case shown="No Error" w1071 {
          tunnel: [w1101 w1103] -> w1088
          tunnel: w1087 -> [w1100 w1103]
          tunnel: w1084 -> [w1099 w1102]
          tunnel: [w1098 w1102] -> w1082
          tunnel: w1079 -> [w1097 _]
          tunnel: w1072 -> [w1096 _]
          frame No Error {
            n480 = call-by-ref "Start Asynchronous Call"(reference=w1099, error in=w1100, "Caller VI Refnum (Callee's Caller)"=w1097, "Inverter v2"=w1096) -> (reference out=w1098:refnum<vi>, error out=w1101:errorcluster)  [unwired: 10 in]
          }
          frame Error {
          }
        }
        n481 = Merge Errors(w1071, w1093) -> (w1090:errorcluster)
        n482 = Close Reference(reference=w1082, error in (no error)=w1088) -> (error out=w1089:errorcluster)
        n483 = call <userlib>:"Clear All Errors__ogtk.vi"("Error In"=w1089) -> ()  [unwired: 3 in, 1 out]
        n484 = call <vilib>:"Add State(s) to Queue__JKI_lib_State_Machine.vi"("State(s) in (\"\")"=w1095) -> ("States Out"=w1094:string)  [unwired: 14 in]
      }
      frame "Action: Stop Daq & Logging" {
        n485 = Unbundle By Name(w1124) -> ("TDMS Enabled"=w1120:bool, "Dependency.Log_Engine"=w1121:refnum<class "Log_Engine.lvclass">, "LoggingEnabled"=w1111:bool, "Dependency.DAQ"=w1123:refnum<class "DAQ_Engine.lvclass">, "DAQEnabled"=w1122:bool)
        n486 = Not(x=w1120) -> (.not. x?=w1119:bool)
        n487 = call "CMD StopLog.vi"("error in (no error)"=w1104, "bypass (F)"=w1119, "Log_Engine in"=w1121) -> ("error out"=w1106:errorcluster, "Log_Engine out"=w1114:refnum<class "Log_Engine.lvclass">)  [unwired: 7 in]
        n488 = Not(x=w1111) -> (.not. x?=w1110:bool)
        n489 = Select(t=u32 0, s=w1119, f=u32 2000 ("milliseconds to wait")) -> (s? t:f=w1116:u32)
        n490 = call <userlib>:"Wait (ms)__ogtk.vi"("error in (no error)"=w1106, "milliseconds to wait"=w1116) -> ("error out"=w1115:errorcluster)  [unwired: 8 in, 1 out]
        n491 = Select(t=u32 0, s=w1110, f=u32 1000 ("milliseconds to wait")) -> (s? t:f=w1108:u32)
        n492 = call "CMD StopESRLog.vi"("error in (no error)"=w1115, "bypass (F)"=w1110, "Log_Engine in"=w1114) -> ("error out"=w1109:errorcluster)  [unwired: 7 in, 1 out]
        n493 = call <userlib>:"Wait (ms)__ogtk.vi"("error in (no error)"=w1109, "milliseconds to wait"=w1108) -> ("error out"=w1107:errorcluster)  [unwired: 8 in, 1 out]
        n494 = case shown="True" w1122 {
          tunnel: w1123 -> [_ w1134]
          tunnel: w1107 -> [w1128 w1132]
          tunnel: [w1128 w1129] -> w1105
          frame False {
          }
          frame True {
            n495 = call "CMD StartStopDAQ.vi"("error in (no error)"=w1132, "DAQEnable"=FALSE, "DAQ_Engine in"=w1134) -> ("error out"=w1131:errorcluster)  [unwired: 7 in, 1 out]
            n496 = call <userlib>:"Wait (ms)__ogtk.vi"("error in (no error)"=w1131, "milliseconds to wait"=u32 1000) -> ("error out"=w1129:errorcluster)  [unwired: 8 in, 1 out]
          }
        }
        n497 = call <vilib>:"Add State(s) to Queue__JKI_lib_State_Machine.vi"("State(s) in (\"\")"=w1127) -> ("States Out"=w1126:string)  [unwired: 14 in]
      }
      frame "Action: SendParamsToProcess" {
        # "This should work, but has not been tested yet"
        n498 = local read "UseDummyVrms"() -> (w1142:bool)
        n499 = Unbundle By Name(w1147) -> ("Self Reference"=w1146:refnum<class "Main.lvclass">)
        n500 = local read "Dummy Vrms"() -> (w1143:dbl)
        n501 = local read "Signal scaling"() -> (w1145:T3[])
        n502 = local read "ESR scaling"() -> (w1135:T7[])
        n503 = To Variant(anything=w1145) -> (Variant=w1144:variant)
        n504 = To Variant(anything=w1142) -> (Variant=w1141:variant)
        n505 = To Variant(anything=w1143) -> (Variant=w1140:variant)
        n506 = To Variant(anything=w1135) -> (Variant=w1139:variant)
        n507 = Build Array(w1144, w1141, w1140, w1139) -> (w1138:variant[])
        n508 = for {
          tunnel: w1146 -> [w1156]
          shift-right: [w1154] -> w1137
          shift-left: w1136 -> [w1152]
          tunnel: w1138 -> [w1151] mode=indexing
          n509 = call "Fire UpdateControlValue Event.vi"("error in (no error)"=w1152, "vData"=w1151, "Main in"=w1156) -> ("error out"=w1155:errorcluster)  [unwired: 7 in, 1 out]
          n510 = call <userlib>:"Wait (ms)__ogtk.vi"("error in (no error)"=w1155, "milliseconds to wait"=u32 500) -> ("error out"=w1154:errorcluster)  [unwired: 8 in, 1 out]
        }
        n511 = call <vilib>:"Add State(s) to Queue__JKI_lib_State_Machine.vi"("State(s) in (\"\")"=w1150) -> ("States Out"=w1149:string)  [unwired: 14 in]
      }
      frame "Action: Shutdown System" {
        # "delay to ensure shutdown status messages\ncan be read in the UI"
        n512 = Unbundle By Name(w1164) -> ("StatusMsg Ref"=w1161:refnum<vi>, "AppTerminateEv"=w1163:refnum<user-event>)
        n513 = call "Fire StopProcess Event.vi"("error in (no error)"=w1157, "Event in"=w1163) -> ("error out"=w1158:errorcluster)  [unwired: 6 in, 3 out]
        n514 = call <userlib>:"Wait (ms)__ogtk.vi"("error in (no error)"=w1158, "milliseconds to wait"=u32 4500) -> ("error out"=w1159:errorcluster)  [unwired: 8 in, 1 out]
        n515 = call <vilib>:"format status message v2.vi"("status msg"="Shutting down Main UI", "Str Refnum"=w1161) -> ()  [unwired: 5 in, 5 out]
        n516 = disable-structure shown="Disabled" {
          frame Disabled {
            n517 = Generate User Event(event data cluster=refnum<notifier> refnum ("event data")) -> ()  [unwired: 3 in, 2 out]
          }
          frame Enabled {
          }
        }
        n518 = call <vilib>:"Add State(s) to Queue__JKI_lib_State_Machine.vi"("State(s) in (\"\")"=w1167) -> ("States Out"=w1166:string)  [unwired: 14 in]
      }
      frame "Action: Wait" {
        n519 = Scan From String(format string="%d", input string=w1169, error in=w1171, default 1=u32 0) -> (error out=w1175:errorcluster, output 1=w1174:u32)  [unwired: 1 in, 2 out]
        n520 = call <userlib>:"Wait (ms)__ogtk.vi"("error in (no error)"=w1175, "milliseconds to wait"=w1174) -> ("error out"=w1170:errorcluster)  [unwired: 8 in, 1 out]
        n521 = call <vilib>:"Add State(s) to Queue__JKI_lib_State_Machine.vi"("State(s) in (\"\")"=w1179) -> ("States Out"=w1178:string)  [unwired: 14 in]
      }
      frame "Action: Terminate AsyncLoop" {
        n522 = Unbundle By Name(w1185) -> ("SMQ"=w1184:refnum<queue>)
        n523 = Flush Queue(queue=w1184) -> (queue out=w1183:refnum<queue>)  [unwired: 1 in, 2 out]
        n524 = call <vilib>:"Add State to Queue with vData.vi"("queue in"=w1183, "state in"="Macro: Exit", "error in"=w1181) -> ("error out"=w1180:errorcluster)  [unwired: 9 in, 3 out]
        n525 = call <vilib>:"Add State(s) to Queue__JKI_lib_State_Machine.vi"("State(s) in (\"\")"=w1188) -> ("States Out"=w1187:string)  [unwired: 14 in]
      }
    }
  }
  n526 = Merge Errors(w3, w2) -> ()  [unwired: 1 out]
